vi "运维调试_总氮.vi"() -> ()   [LabVIEW 2016, in "总氮.lvlib"]
uses:
  <vilib>/Platform/TimedLoop/XDataNode/timing_clust.ctl
  <vilib>/Platform/TimedLoop/XDataNode/nitl_modes.ctl
  <vilib>/Platform/TimedLoop/XDataNode/wakeup.ctl
  <vilib>/Utility/miscctls.llb/LVPointTypeDef.ctl
  <vilib>/Platform/TimedLoop/XDataNode/XDataNode.xnode
  <vilib>/Platform/TimedLoop/XDataNode/XDNodeRunTimeDep.lvlib
  <vilib>/Utility/config.llb/NI_LVConfig.lvlib
panel:
  in  "总氮自动测试量程配置":T1
  out "温度2":sgl
  out "温度1":sgl
  out "ADC":sgl
  out "字符串":string
  out "固件版本号":string
  in  "数组":string[](array[string])
  in  "备用系数写入":bool
  in  "备用系数读取":bool
  in  "备用系数":T2
  in  "量程切换阈值写入":bool
  in  "量程切换阈值读取":bool
  in  "量程切换阈值":cluster{"阈值":dbl, "标液浓度":dbl}
  in  "参数下拉列表":enum16{"总磷", "总氮"}(ring)=enum."总氮"
  in  "量程下拉列表":enum16{"低量程", "高量程"}(ring)
  in  "测量模式下拉列表":enum16{"水样测量", "空白核查", "跨度核查", "标样核查", "加标回收"}(ring)
  in  "公式":cluster{"X^2":dbl, "X":dbl, "b":dbl}
  in  "写公式":bool
  in  "读公式":bool
  in  "精度":dbl=4.0
  in  "样品5 F0":dbl
  in  "样品5 F1":dbl
  in  "样品4 F1":dbl
  in  "样品4 F0":dbl
  in  "样品3 F0":dbl
  in  "样品3 F1":dbl
  in  "样品2 F0":dbl
  in  "样品2 F1":dbl
  in  "样品1 F1":dbl
  in  "样品1 F0":dbl
  in  "method":u16(ring) items=["最小二乘", "最小绝对残差", "Bisquare"]
  in  "模型":enum32{"线性", "多项式"}(ring)
  out "r^2":dbl format="%.7g"
  out "拟合公式":string
  in  "样品2启用":bool
  in  "样品5启用":bool
  in  "样品4启用":bool
  in  "样品3启用":bool
  in  "样品1启用":bool
  in  "标液浓度5":dbl
  out "测量吸光度5":dbl
  in  "标液浓度4":dbl
  out "测量吸光度4":dbl
  in  "标液浓度3":dbl
  out "测量吸光度3":dbl
  in  "标液浓度2":dbl
  out "测量吸光度2":dbl
  out "测量吸光度1":dbl
  in  "标液浓度1":dbl
  out "XY图":cluster{"X Values":dbl[], "Y Values":dbl[]}[](graph)
  in  "返回":bool
  in  "设置":bool
  out "序列号":string="序列号"
  out "总氮测量数据":T3(xcontrol)
  out "集成报警信息":string
  out "设置值":dbl
  out "定时启动":bool
  out "总磷总氮运行状态":T4(xcontrol)
  in  "停止":bool
  in  "手动启动":bool
  in  "单步测试":bool
  in  "总磷氨氮调试":u16[](xcontrol)
  out "F3":sgl format="%#.6f"
  out "F2":sgl format="%#.6f"
  out "F1":sgl format="%#.6f"
  out "F0":sgl format="%#.6f"
  out "多列列表框":i32(listbox)
  # "COM10"
  # "参数设置"
  # "标液浓度"
  # "F0"
  # "F1"
  # "吸光值显示"
  # "样品一"
  # "辅\n助\n计\n算\n区"
  # "样品二"
  # "样品三"
  # "样品四"
  # "样品五"
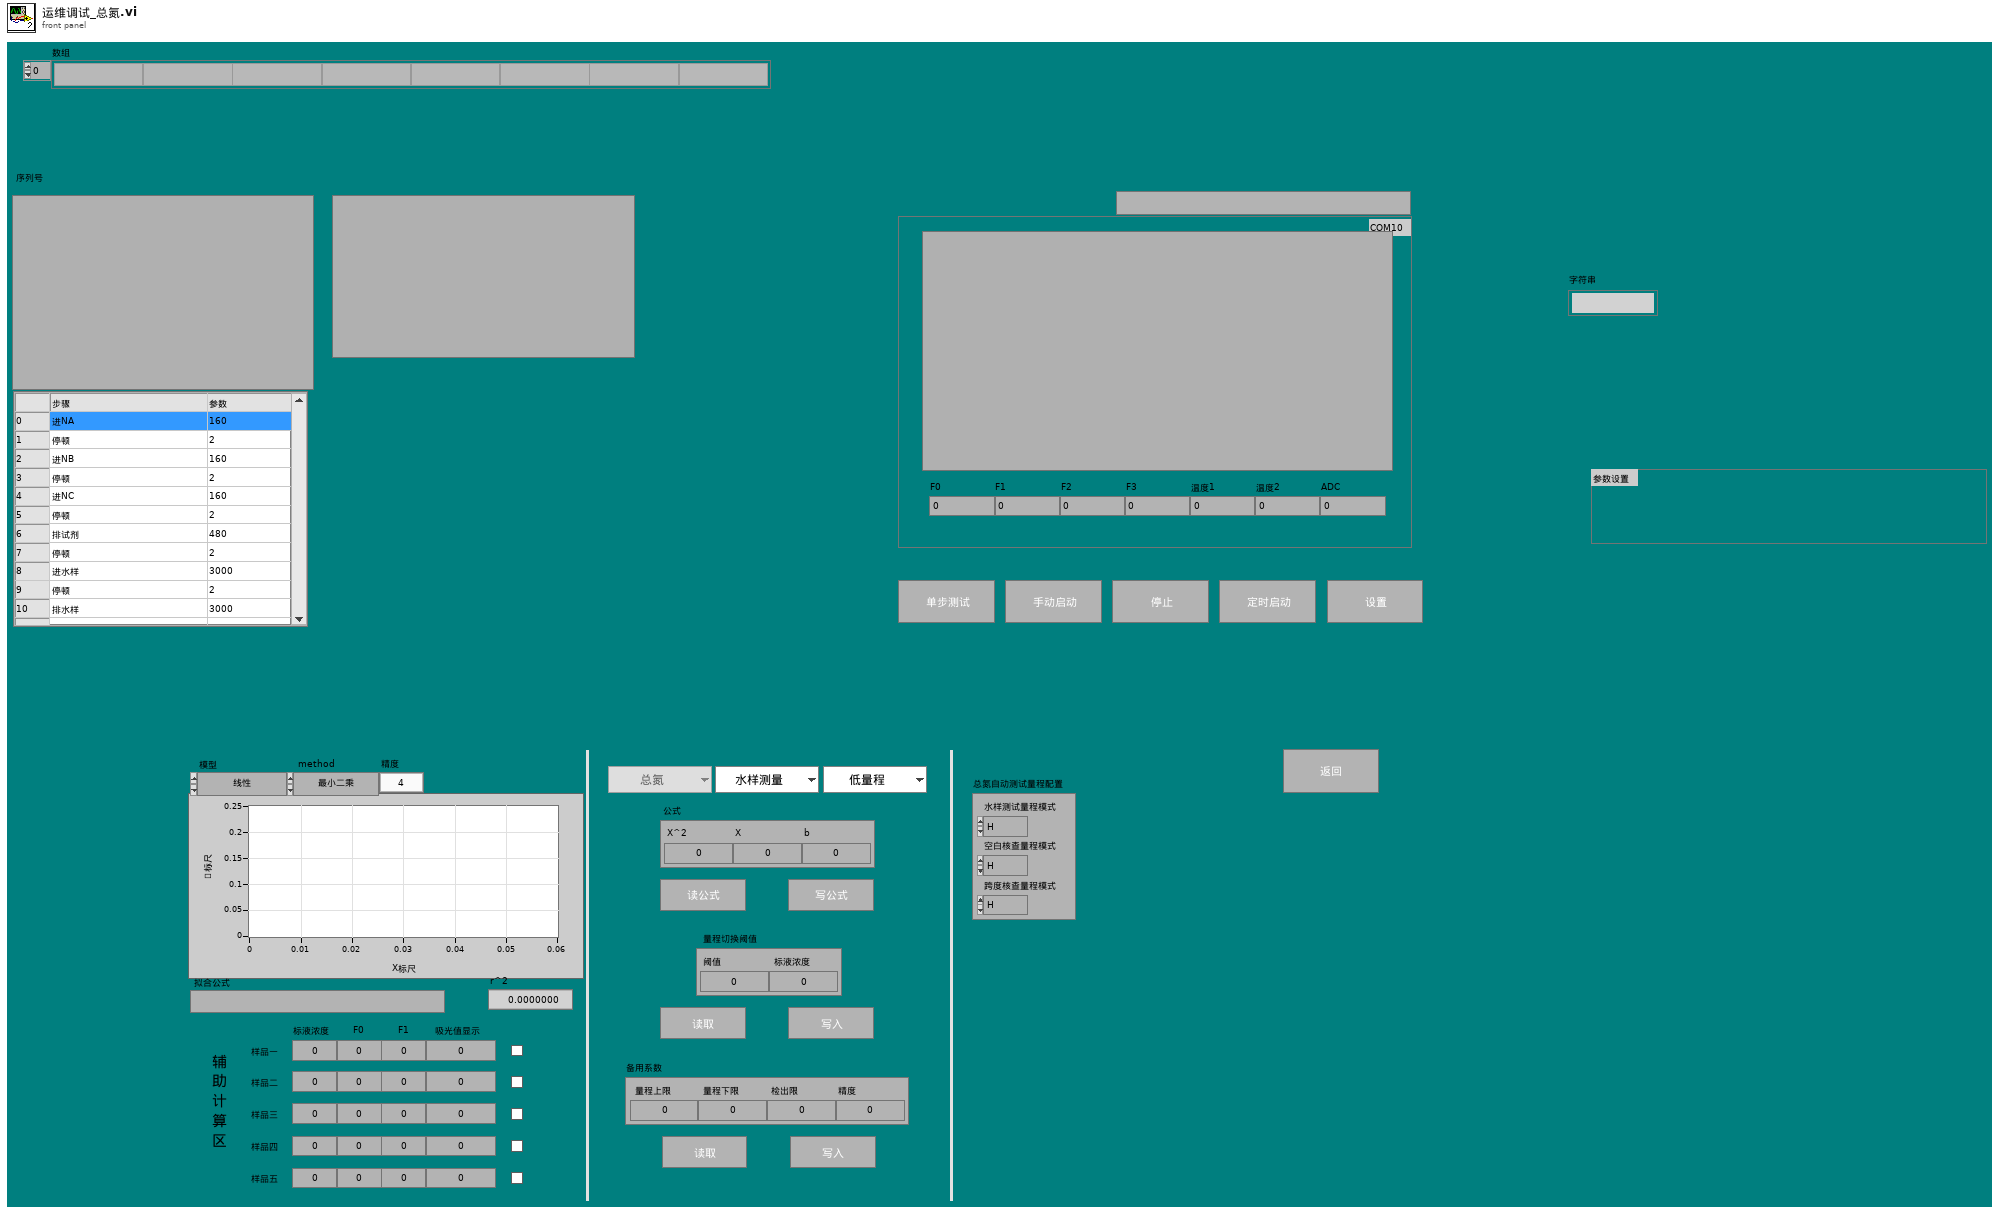
[diagram p1: front panel]
types:
  T1 = cluster{"水样测试量程模式":enum16{"H", "L", "AUTO"}, "空白核查量程模式":enum16{"H", "L", "AUTO"}, "跨度核查量程模式":enum16{"H", "L", "AUTO"}}
  T2 = cluster{"量程上限":dbl, "量程下限":dbl, "检出限":dbl, "精度":dbl}
  T3 = cluster{"flowid":u16, "测量精度":u16, "测量数据区":cluster{"因子编码":u32, "单位":u16, "标样参考值":sgl, "水样数据时间":timestamp, "水样实测值":sgl, "水样数据标识":string, "标样数据时间":timestamp, "标样实测值":sgl, "标样数据标识":string, "空白数据时间":timestamp, "空白实测值":sgl, "空白数据标识":string, "零点核查数据时间":timestamp, "零点核查实测值":sgl, "零点核查数据标识":string, "跨度核查数据时间":timestamp, "跨度核查实测值":sgl, "跨度核查数据标识":string, "加标回收数据时间":timestamp, "加标回收实测值":sgl, "加标回收数据标识":string, "平行样数据时间":timestamp, "平行样实测值":sgl, "平行样数据标识":string, "F0":sgl, "F1":sgl, "F2":sgl, "F3":sgl, "F4":sgl, "F5":sgl, "F6":sgl, "F7":sgl, "温度":sgl, "湿度":sgl, "X值":sgl}}
  T4 = cluster{"系统时间":timestamp, "工作状态":enum16{"空闲", "水样测试", "标样核查", "零点核查", "跨度核查", "空白测试", "平行样测试", "加标回收", "空白校准", "标样校准", "初始化（清洗）"}, "测量模式":enum16{"待机", "连续模式", "周期模式", "定点模式", "受控模式", "手动模式"}, "告警代码":enum16{"无告警", "缺试剂告警", "缺水样告警", "缺蒸馏水告警", "缺标液告警", "仪表漏液告警", "标定异常告警", "超量程告警", "加热异常", "低试剂预警", "超上限告警", "超下限告警", "仪表内部其他异常", "滴定异常告警", "电极异常告警", "量程切换告警", "参数设置告警", "PH电极电位异常", "电导率电极异常", "浊度光度异常", "溶解氧电极异常", "溶解氧光强异常", "温度异常告警", "PH异常告警", "溶解氧异常告警", "电导率异常告警", "浊度异常告警", "叶绿素异常告警", "藻密度异常告警", "蓝绿藻异常告警", "ORP异常告警", "氨氮异常告警", "清洁刷异常告警", "SD卡异常告警", "蓝牙异常告警", "Wifi异常告警", "流程异常告警"}, "故障代码":enum16{"无故障", "电机故障", "温度故障", "通讯故障", "滴定故障"}, "日志代码":u16, "软件版本":u16, "F0":sgl, "F1":sgl, "F2":sgl, "F3":sgl, "T":sgl, "H":sgl, "id":u16, "flowid":u16, "量程":u16, "总磷控温温度1":sgl, "营养盐控温温度2":sgl, "ADC":sgl}
  T5 = typedef "LVPointTypeDef.ctl" = cluster{"Horizontal":i16, "Vertical":i16}
  T6 = cluster{"因子编码":u32, "单位":u16, "标样参考值":sgl, "水样数据时间":timestamp, "水样实测值":sgl, "水样数据标识":string, "标样数据时间":timestamp, "标样实测值":sgl, "标样数据标识":string, "空白数据时间":timestamp, "空白实测值":sgl, "空白数据标识":string, "零点核查数据时间":timestamp, "零点核查实测值":sgl, "零点核查数据标识":string, "跨度核查数据时间":timestamp, "跨度核查实测值":sgl, "跨度核查数据标识":string, "加标回收数据时间":timestamp, "加标回收实测值":sgl, "加标回收数据标识":string, "平行样数据时间":timestamp, "平行样实测值":sgl, "平行样数据标识":string, "F0":sgl, "F1":sgl, "F2":sgl, "F3":sgl, "F4":sgl, "F5":sgl, "F6":sgl, "F7":sgl, "温度":sgl, "湿度":sgl, "X值":sgl}
  T7 = enum16{"空闲", "水样测试", "标样核查", "零点核查", "跨度核查", "空白测试", "平行样测试", "加标回收", "空白校准", "标样校准", "初始化（清洗）"}
  T8 = typedef "XDNodeRunTimeDep.lvlib/timing_clust.ctl" = cluster{"Expected End [f-1]":u64, "Actual End [f-1]":u64, "Finished Late? [f-1]":bool, "Expected End [i-1]":u64, "Actual End [i-1]":u64, "Finished Late? [i-1]":bool, "Expected Start [i]":u64, "Actual Start [i]":u64, "Expected Start [f]":u64, "Actual Start [f]":u64, "Source Name":string, "Structure Name":string, "Period":i64, "Deadline":i64, "Offset":i64, "Start":i64, "Priority":i32, "Timeout":i32, "Mode":T9, "Wakeup Reason":T10, "Error":errorcluster, "Source Type":string, "Secondary Source Type":string, "Global End Time":u64, "Global Start Time":u64, "Frame Duration":u64, "Iteration Duration":u64, "Assigned CPU":i32, "I/O Scan Engine Mode":u32}
  T9 = typedef "XDNodeRunTimeDep.lvlib/nitl_modes.ctl" = enum32{"No Change", "Process missed periods, maintain original phase", "Discard missed periods, maintain original phase", "Process missed periods, ignore original phase", "Discard missed periods, ignore original phase"}
  T10 = typedef "XDNodeRunTimeDep.lvlib/wakeup.ctl" = enum32{"Normal", "Aborted", "Asynchronous wakeup", "Timing source error", "Timed loop error", "Timeout"}
  T11 = cluster{"启动模式":enum16{"标液测量", "水样测量", "零液测量", "盲样测量", "加标回收"}, "启动参数":u16, "量程":enum16{"低量程", "高量程"}}
  T12 = cluster{"时间标识":timestamp, "设备":string, "日志信息":string, "流程参数":string}
  T13 = cluster{"时间标识":timestamp, "设备":string, "日志信息":string}
  T14 = enum16{"无告警", "缺试剂告警", "缺水样告警", "缺蒸馏水告警", "缺标液告警", "仪表漏液告警", "标定异常告警", "超量程告警", "加热异常", "低试剂预警", "超上限告警", "超下限告警", "仪表内部其他异常", "滴定异常告警", "电极异常告警", "量程切换告警", "参数设置告警", "PH电极电位异常", "电导率电极异常", "浊度光度异常", "溶解氧电极异常", "溶解氧光强异常", "温度异常告警", "PH异常告警", "溶解氧异常告警", "电导率异常告警", "浊度异常告警", "叶绿素异常告警", "藻密度异常告警", "蓝绿藻异常告警", "ORP异常告警", "氨氮异常告警", "清洁刷异常告警", "SD卡异常告警", "蓝牙异常告警", "Wifi异常告警", "流程异常告警"}
  T15 = typedef "LVRowAndColumnUnsignedTypeDef.ctl" = cluster{"Row":u32, "Column":u32}
  T16 = cluster{"站号":u16, "量程切换":enum32{"H", "L", "AUTO"}, "控制命令":enum16{"启动测量", "标样核查", "零点核查", "跨度核查", "空白测试", "平行样测试", "加标回收", "空白校准", "标样校准", "初始化（清洗）", "停止测试", "仪器重启", "校时", "模式设置", "测量间隔设置"}, "模式设置":enum16{"待机", "连续模式", "周期模式", "定点模式", "受控模式", "手动模式"}, "测量间隔":u16}
  T17 = typedef "NI_LVConfig.lvlib/Config Data RefNum.ctl" = refnum<k1>
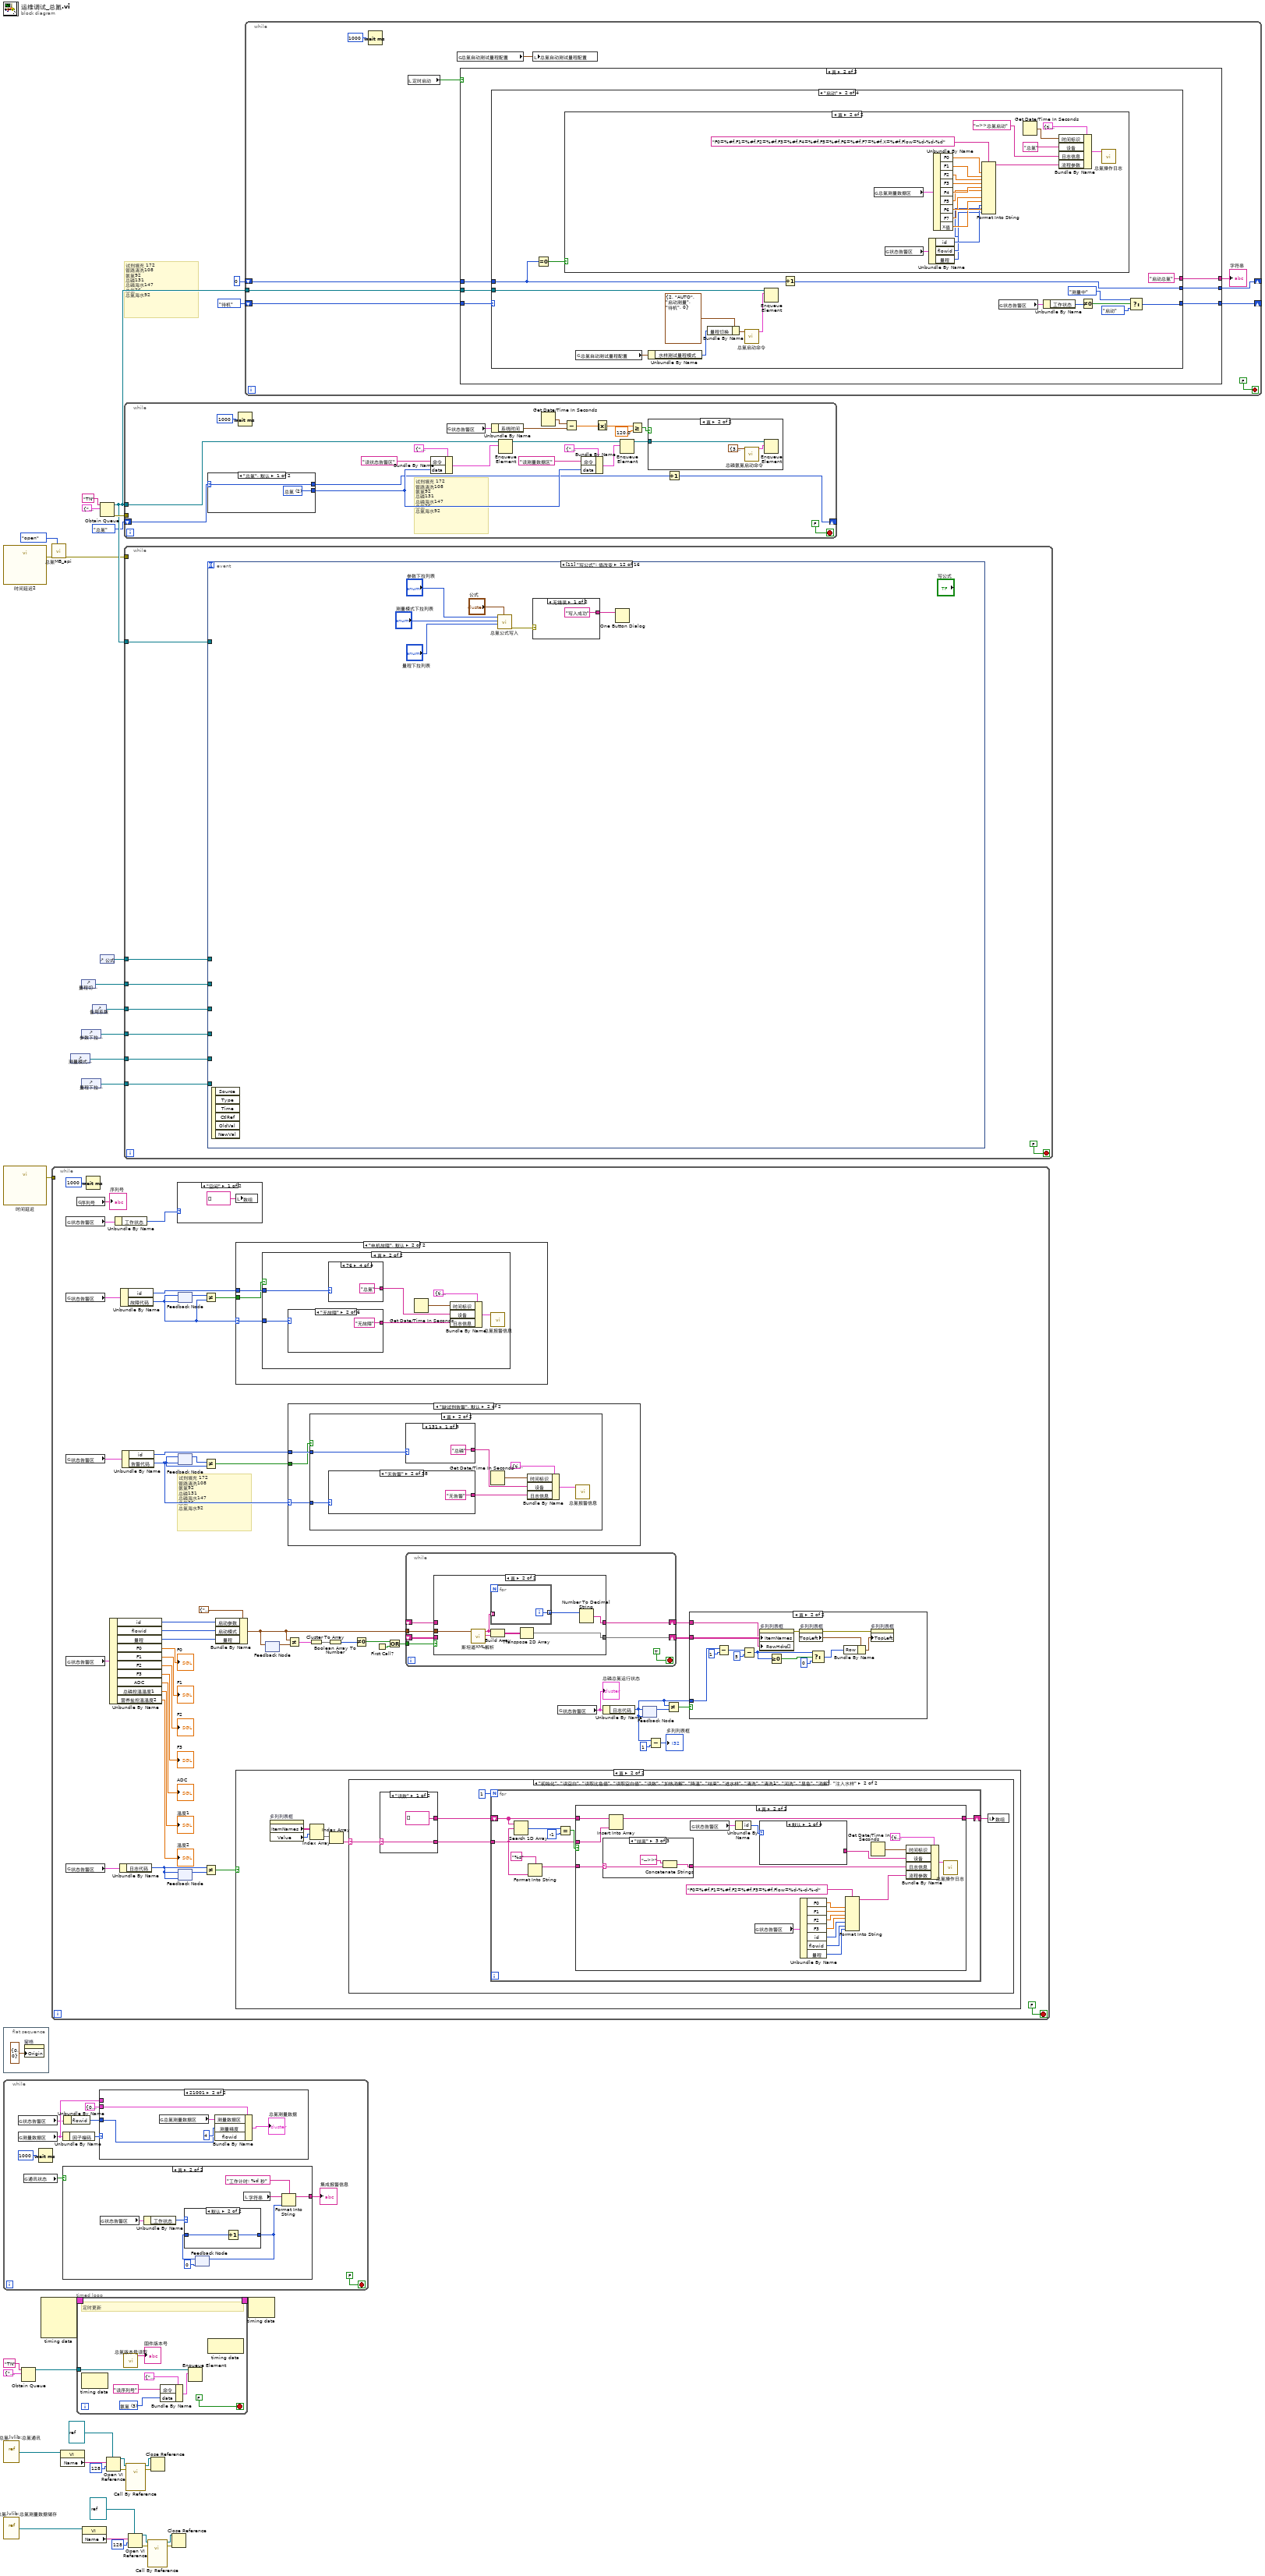
[diagram p0: block diagram]
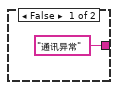
[diagram p2: hidden frame]
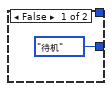
[diagram p5: hidden frame]
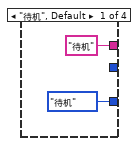
[diagram p6: hidden frame]
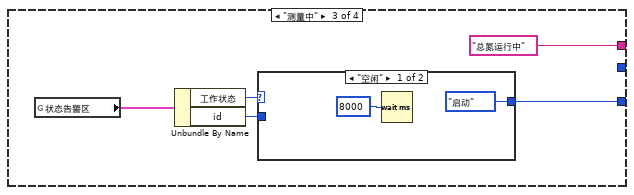
[diagram p8: hidden frame]
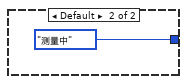
[diagram p9: hidden frame]
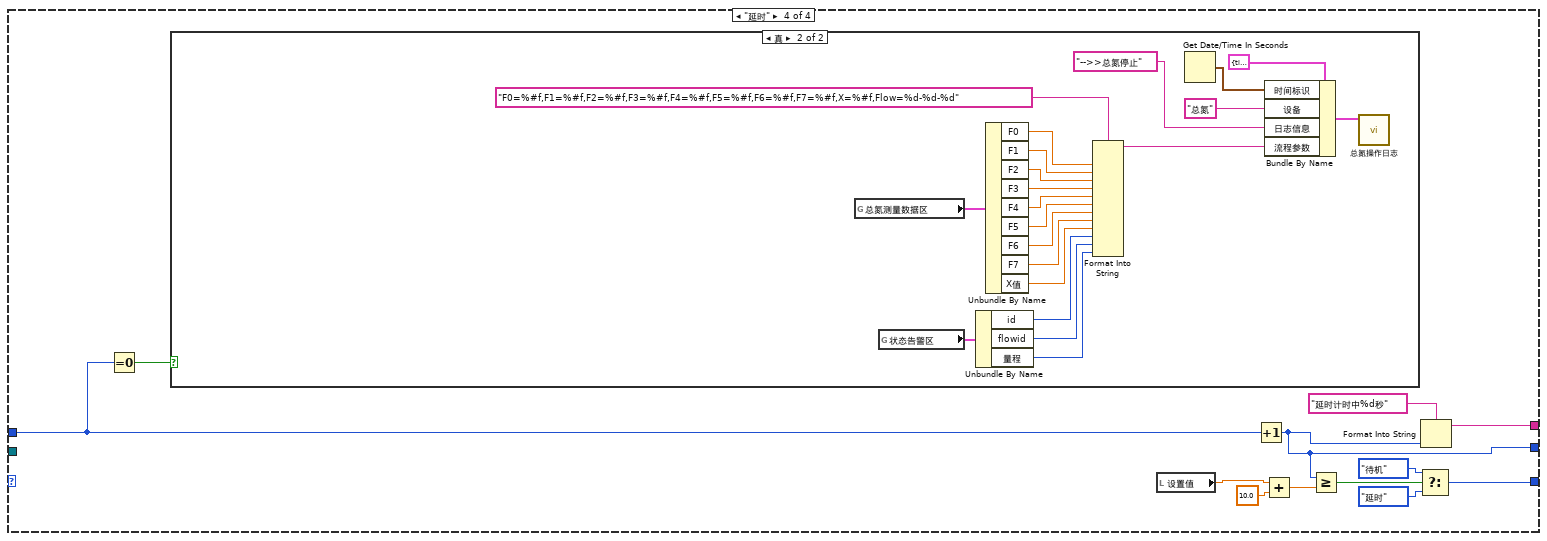
[diagram p10: hidden frame]
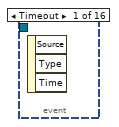
[diagram p12: hidden frame]
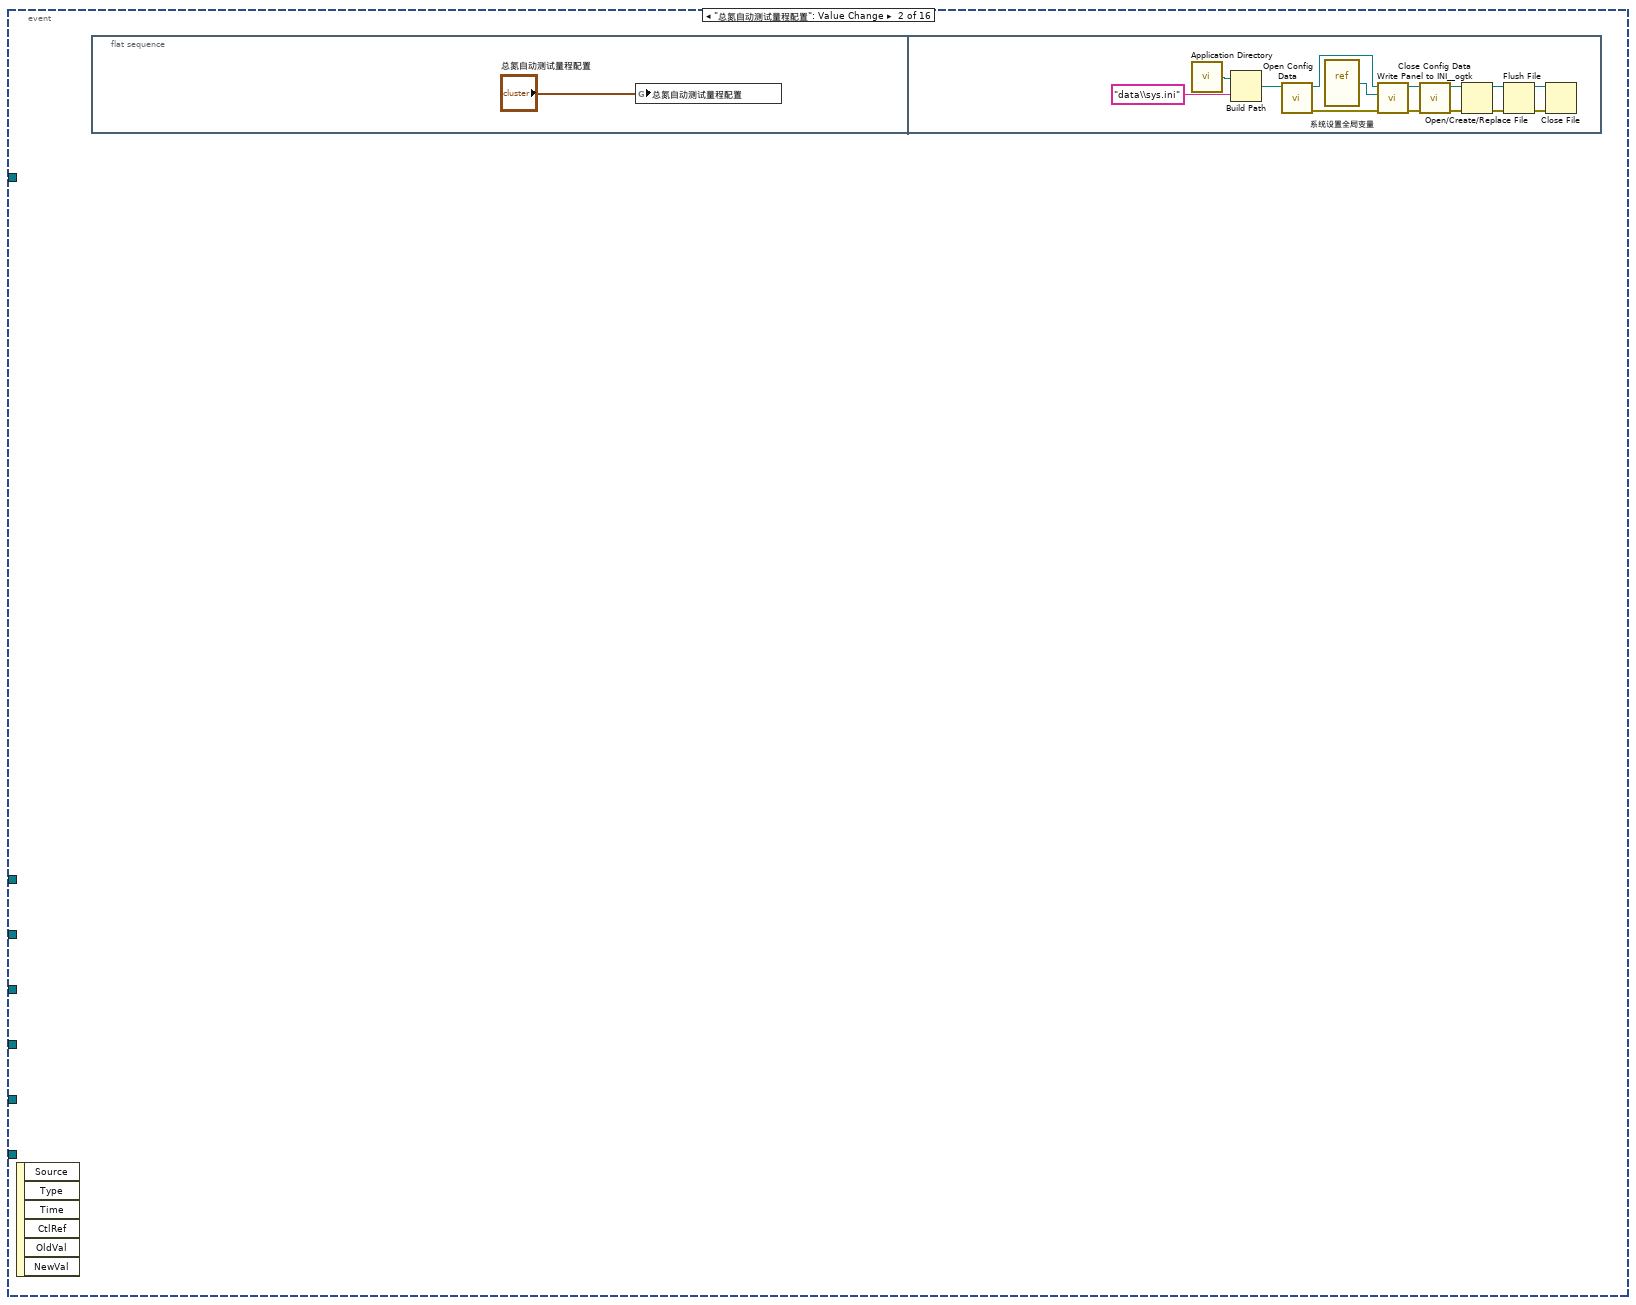
[diagram p13: hidden frame]
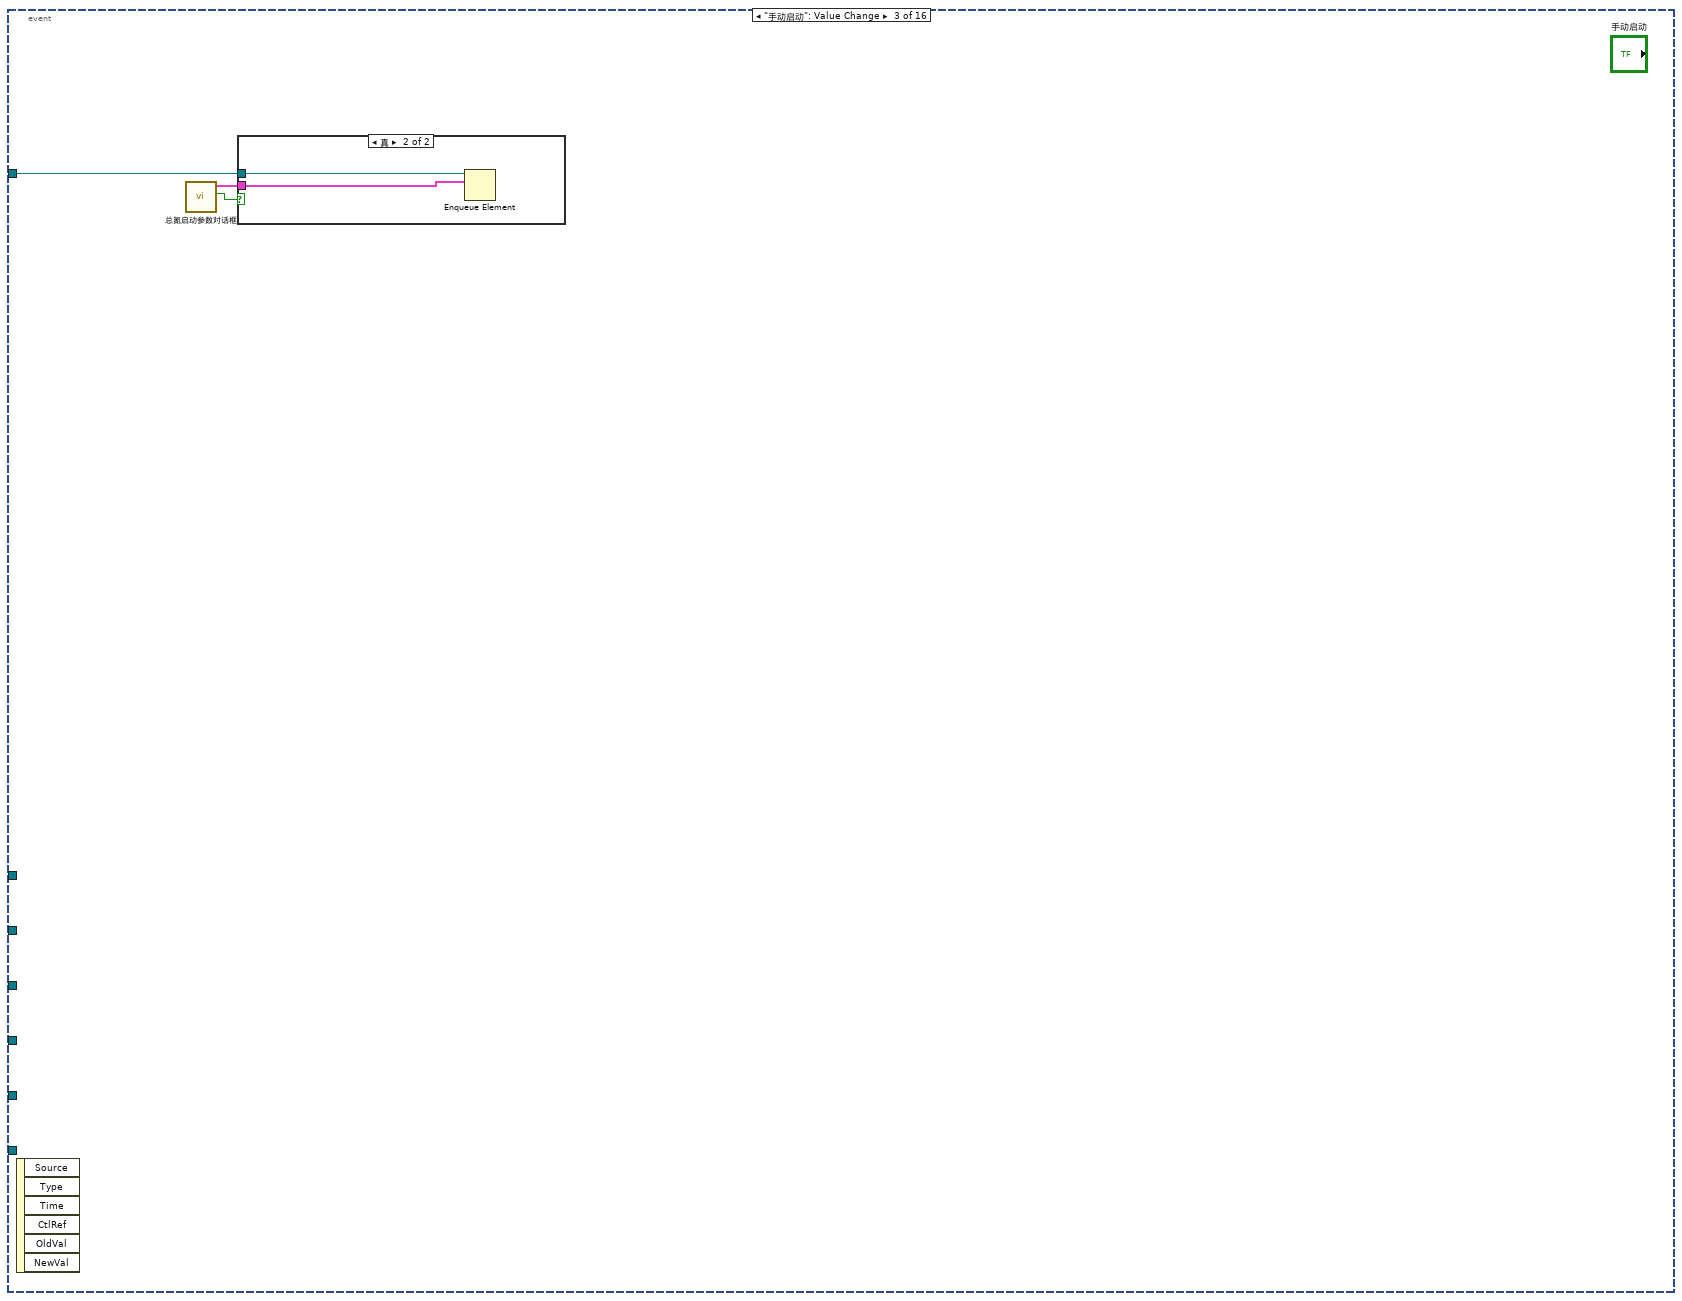
[diagram p14: hidden frame]
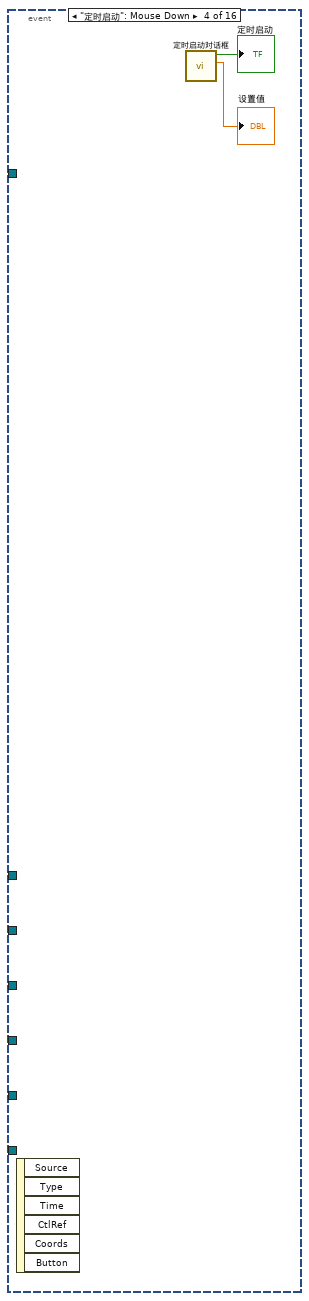
[diagram p16: hidden frame]
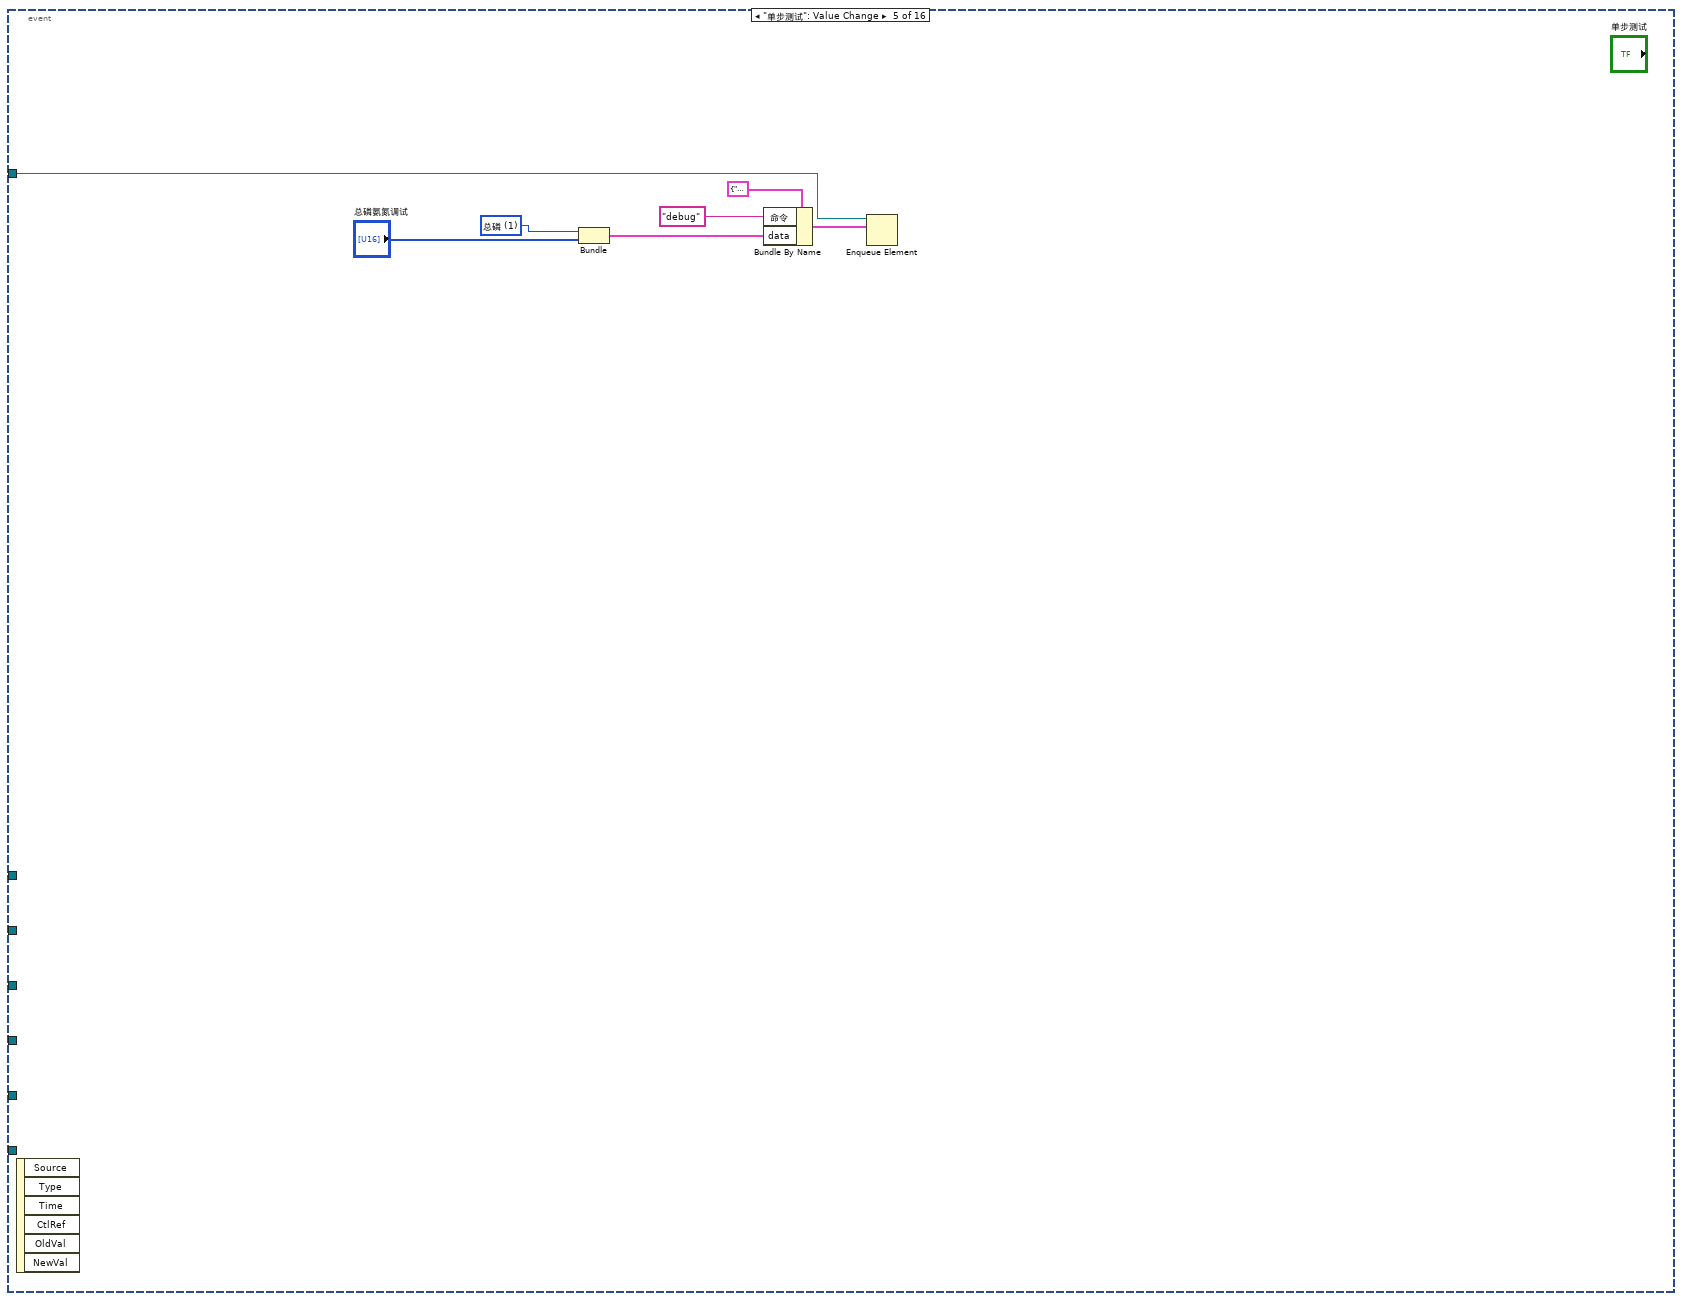
[diagram p17: hidden frame]
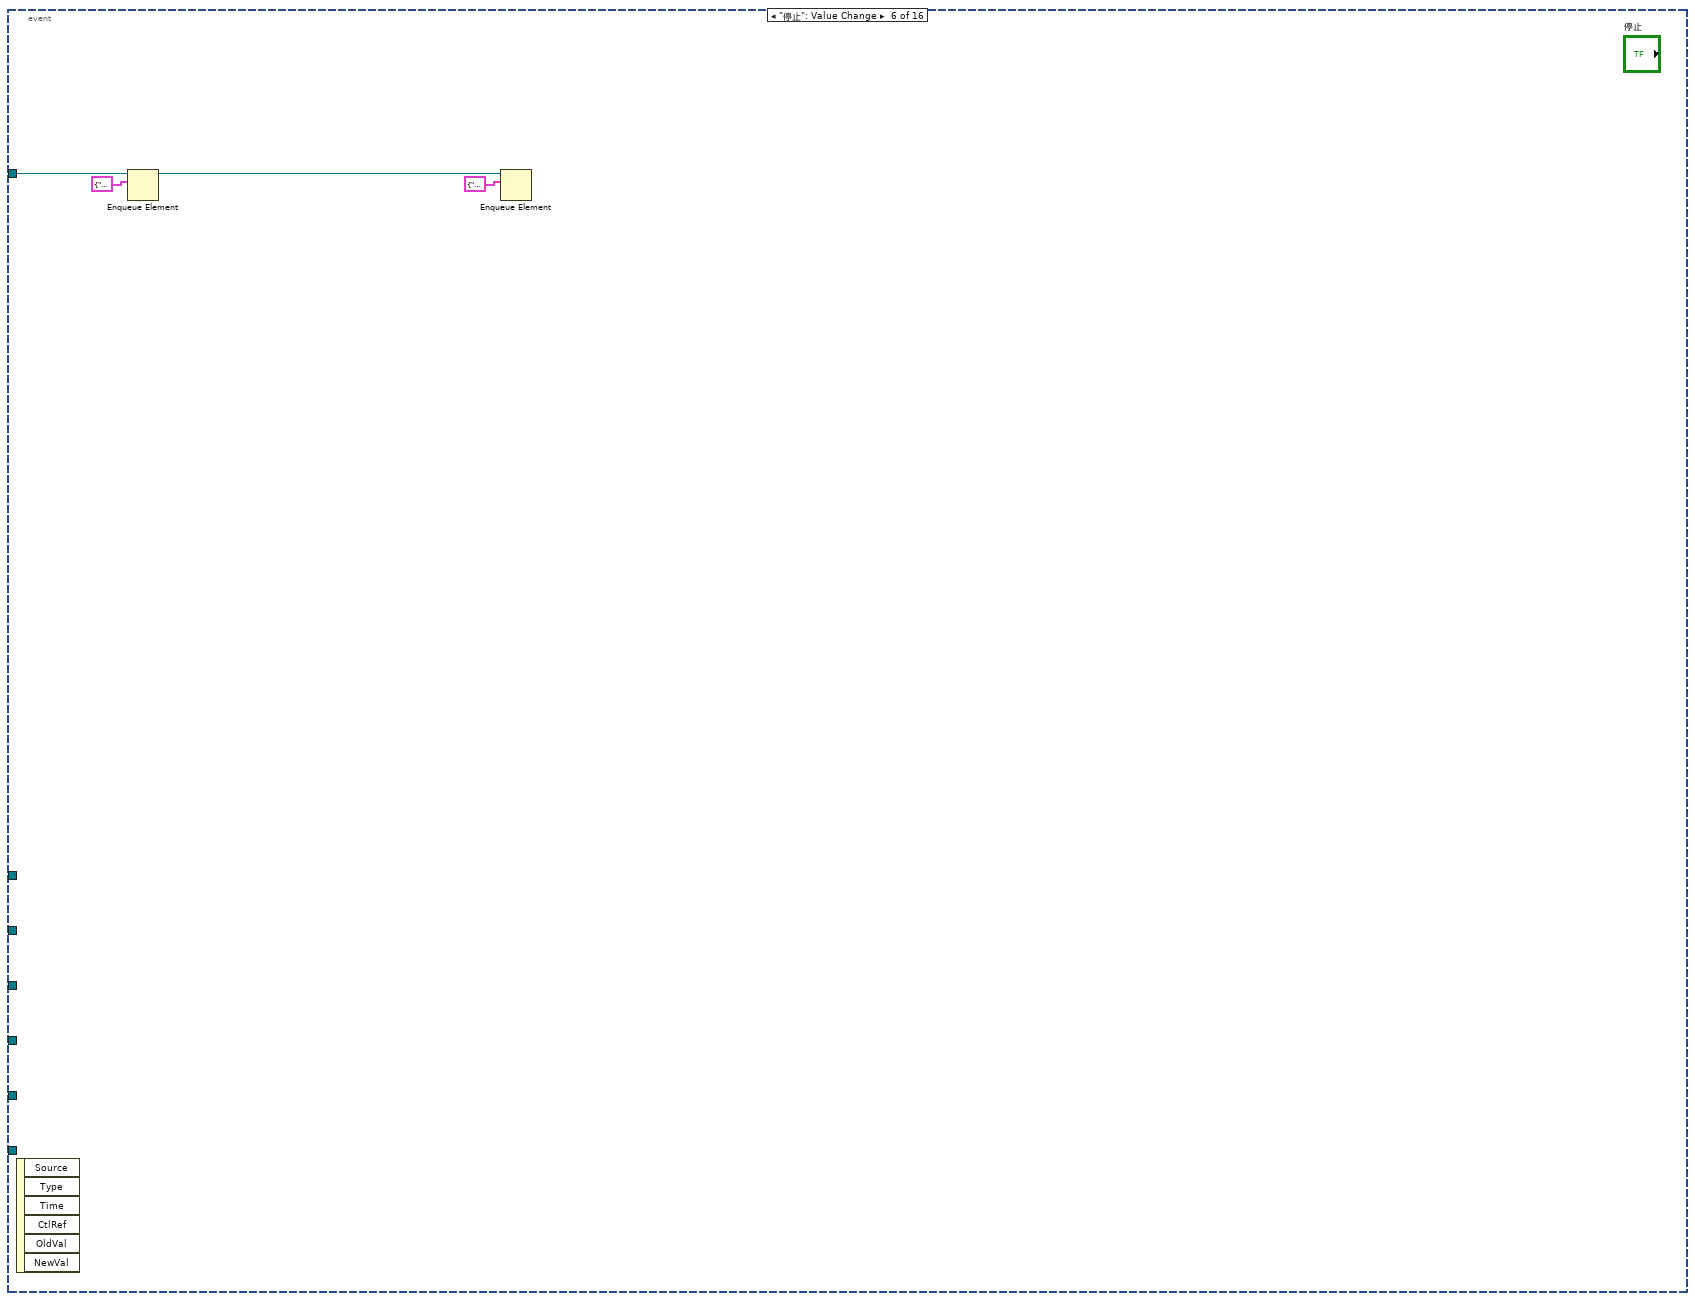
[diagram p18: hidden frame]
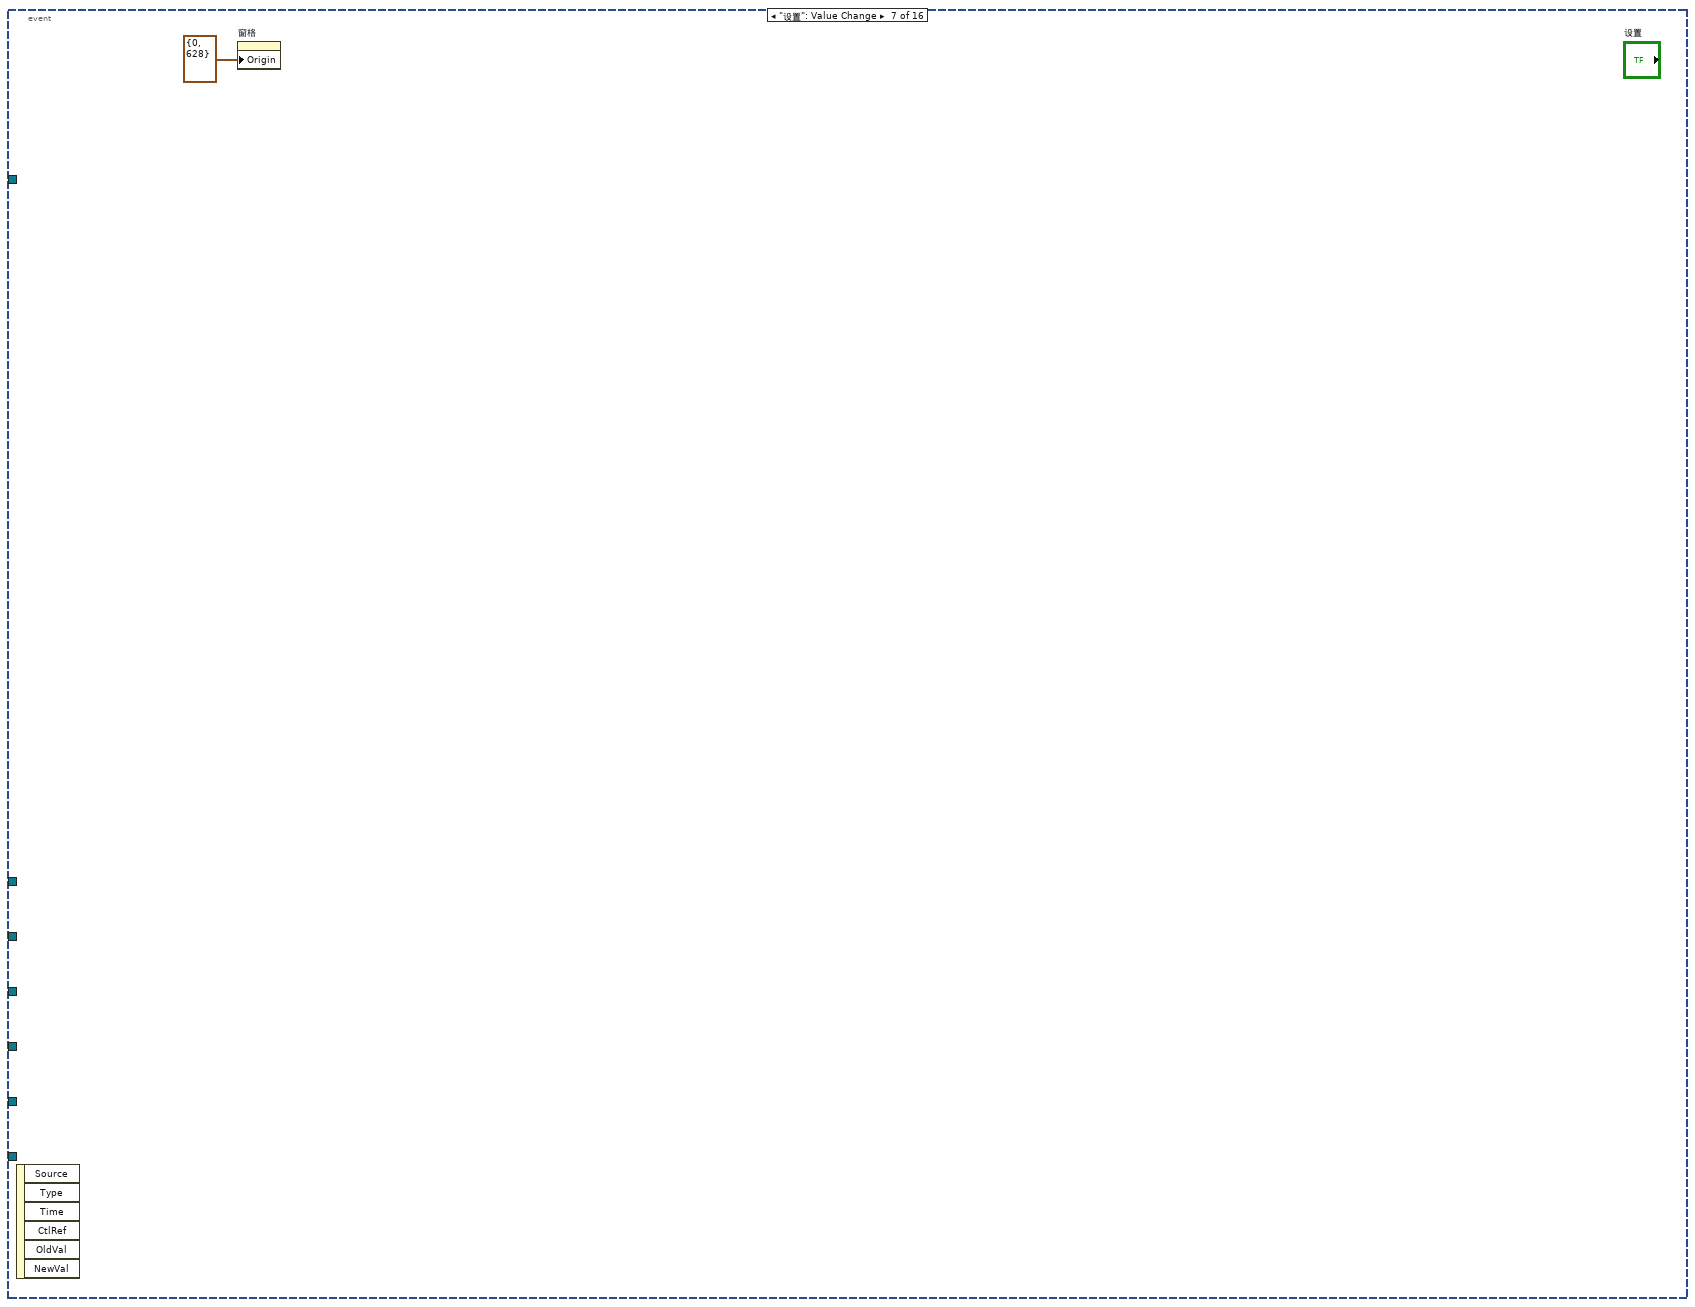
[diagram p19: hidden frame]
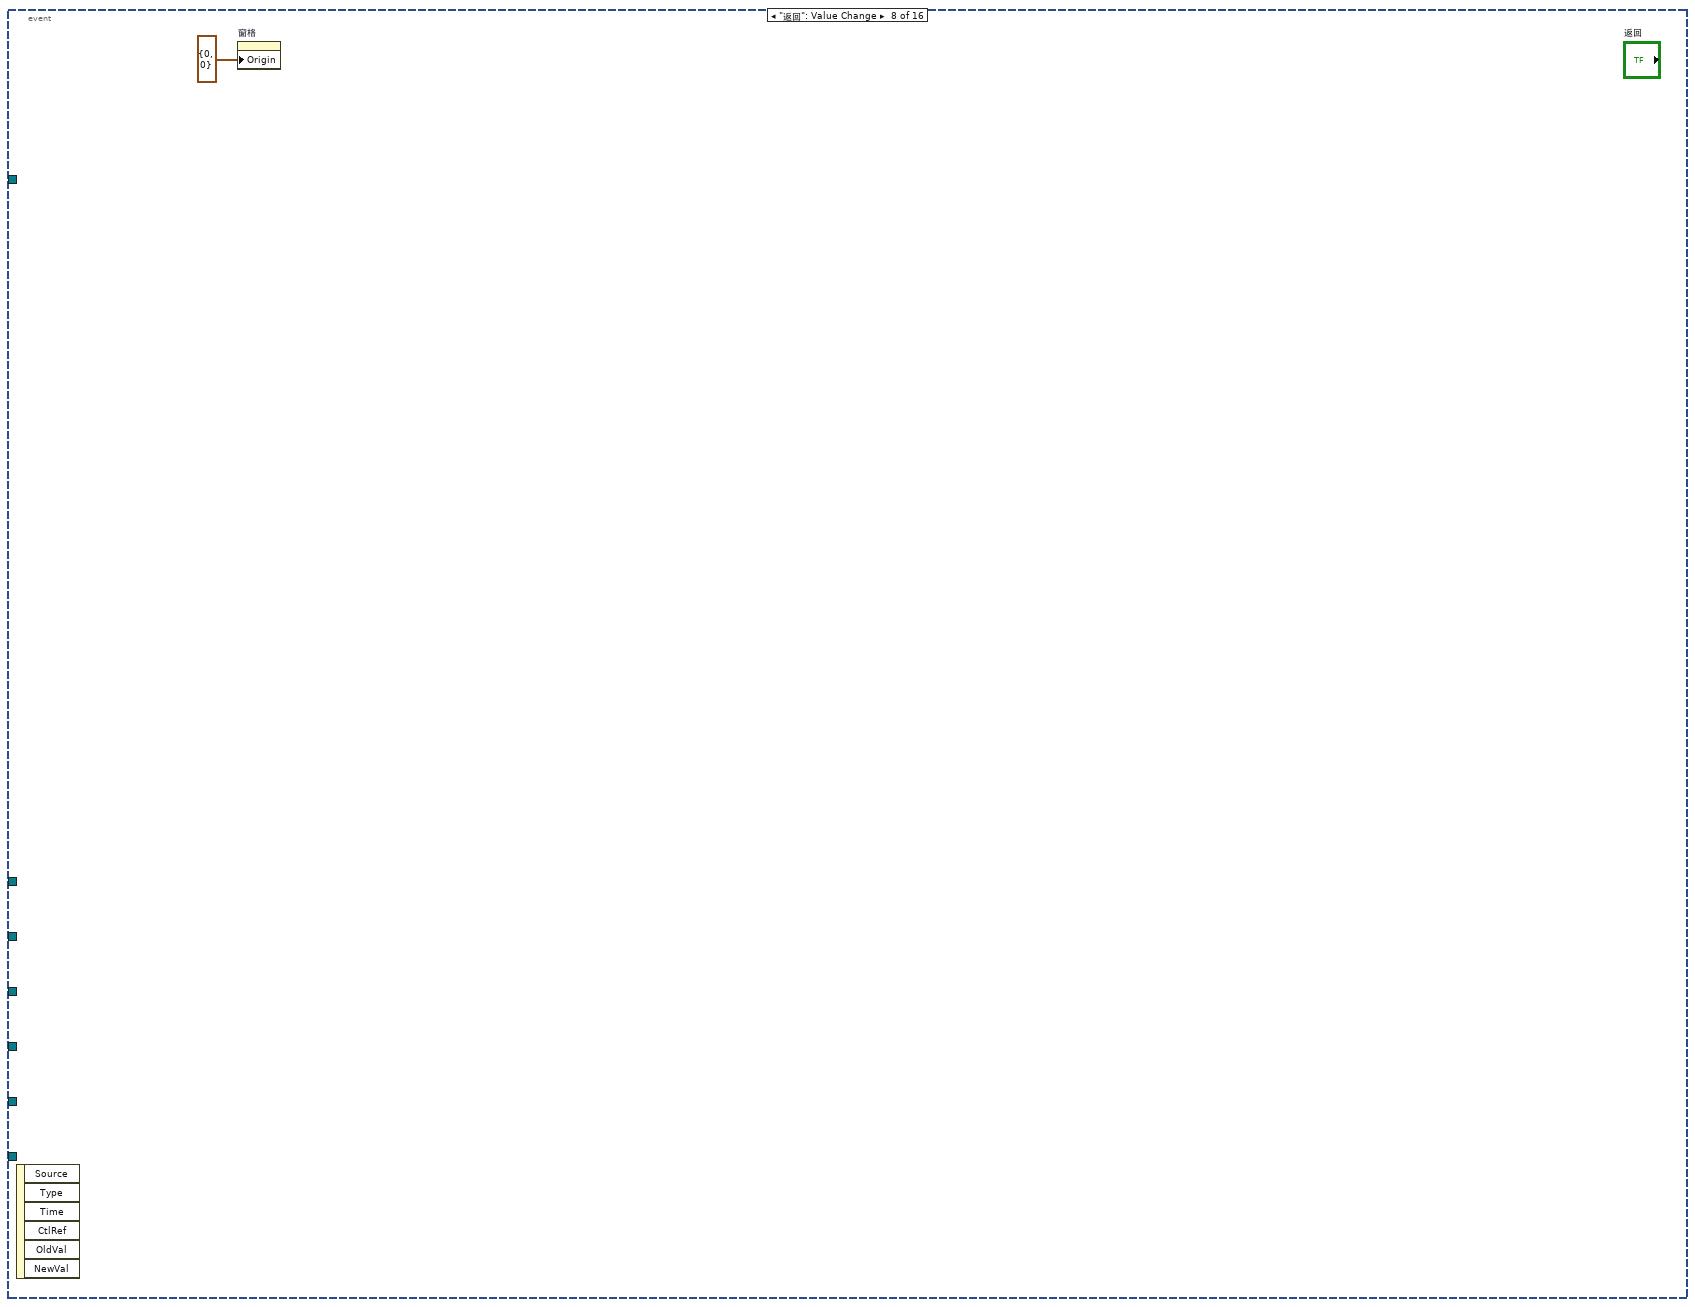
[diagram p20: hidden frame]
diagram:
  # "试剂填充 172 \n管路清洗108\n氨氮92\n总磷131\n总磷海水147\n总氮76\n总氮海水92"
  n1 = call "时间延迟2"() -> ("error out"=w1:errorcluster)  [unwired: 11 in]
  n2 = call "时间延迟"() -> ("error out"=w9:errorcluster)  [unwired: 11 in]
  n3 = flat-sequence {
    frame #0 {
      n4 = property on="窗格" class="Pane"("Origin"=T5 {"Horizontal"=0, "Vertical"=0} ("原点")) -> ()  [unwired: 2 in, 2 out]
    }
  }
  n5 = while {
    stop <- FALSE stop-if-true
    n6 = global read "VAR总氮全局变量.vi" "状态告警区"() -> (w42:T4)
    n7 = global read "VAR总氮全局变量.vi" "测量数据区"() -> (w46:T6)
    n8 = global read "VAR总氮全局变量.vi" "通讯状态"() -> (w44:bool)
    n9 = Wait (ms)(milliseconds to wait=u32 1000 ("等待时间（毫秒）")) -> ()  [unwired: 1 out]
    n10 = Unbundle By Name(w46) -> ("因子编码"=w45:u32)
    n11 = case shown="真" w44 {
      tunnel: ["通讯异常" ("集成报警信息") w51] -> w43
      frame False {
      }
      frame True {
        n12 = global read "VAR总氮全局变量.vi" "状态告警区"() -> (w57:T4)
        n13 = Unbundle By Name(w57) -> ("工作状态"=w56:T7)
        n14 = feedback #1(0) -> (w54:i32)
        n15 = case shown="默认" w56 {
          tunnel: w54 -> [_ w59]
          tunnel: [_ w58] -> w52
          frame "空闲" {
          }
          frame Default {
            n16 = Increment(x=w59) -> (x+1=w58:i32)
          }
        }
        n17 = feedback-in #1(w52) -> ()
        n18 = local read "字符串"() -> (w50:string)
        n19 = Format Into String(format string="工作计时: %d 秒" ("格式字符串"), initial string=w50, w52) -> (resulting string=w51:string)  [unwired: 1 in, 1 out]
      }
    }
    "集成报警信息" <- w43
    n20 = Unbundle By Name(w42) -> ("flowid"=w41:u16)
    n21 = case shown="21001" w45 {
      tunnel: w46 -> [_ _]
      tunnel: w41 -> [_ w63]
      tunnel: T3 {"flowid"=0, "测量精度"=0, "测量数据区"={"因子编码"=0, "单位"=0, "标样参考值"=0.0, "水样数据时间"=timestamp(0 s since 1904-01-01), "水样实测值"=0.0, "水样数据标识"="", "标样数据时间"=timestamp(0 s since 1904-01-01), "标样实测值"=0.0, "标样数据标识"="", "空白数据时间"=timestamp(0 s since 1904-01-01), "空白实测值"=0.0, "空白数据标识"="", "零点核查数据时间"=timestamp(0 s since 1904-01-01), "零点核查实测值"=0.0, "零点核查数据标识"="", "跨度核查数据时间"=timestamp(0 s since 1904-01-01), "跨度核查实测值"=0.0, "跨度核查数据标识"="", "加标回收数据时间"=timestamp(0 s since 1904-01-01), "加标回收实测值"=0.0, "加标回收数据标识"="", "平行样数据时间"=timestamp(0 s since 1904-01-01), "平行样实测值"=0.0, "平行样数据标识"="", "F0"=0.0, "F1"=0.0, "F2"=0.0, "F3"=0.0, "F4"=0.0, "F5"=0.0, "F6"=0.0, "F7"=0.0, "温度"=0.0, "湿度"=0.0, "X值"=0.0}} ("总氮测量数据") -> [_ w62]
      frame Default {
      }
      frame 21001 {
        n22 = global read "VAR总氮全局变量.vi" "总氮测量数据区"() -> (w61:T6)
        n23 = Bundle By Name(cluster=w62, "测量数据区"=w61, "测量精度"=u16 4, "flowid"=w63) -> (→"总氮测量数据":T3)
      }
    }
  }
  n24 = vi-ref "总氮.lvlib:总氮通讯.vi"() -> (w32:refnum<vi>)
  n25 = vi-ref "总氮.lvlib:总氮测量数据储存.vi"() -> (w24:refnum<vi>)
  n26 = Obtain Queue(name (unnamed)="TN" ("名称（未命名）"), element data type=cluster{"命令":string, "data":variant} {"命令"="", "data"=variant}) -> (queue out=w2:refnum<queue>)  [unwired: 3 in, 2 out]
  n27 = node-c288() -> (w6:T8)  [unwired: 4 in]
  n28 = call "总氮MB_api.vi"("STEP"=enum16{"open", "read", "write", "close"}."open", "Error in"=w1) -> ("error out"=w8:errorcluster)  [unwired: 7 in, 2 out]
  n29 = while {
    tunnel: w9 -> [_]
    stop <- FALSE stop-if-true
    # "试剂填充 172 \n管路清洗108\n氨氮92\n总磷131\n总磷海水147\n总氮76\n总氮海水92"
    n30 = global read "VAR总氮全局变量.vi" "状态告警区"() -> (w76:T4)
    n31 = global read "VAR总氮全局变量.vi" "状态告警区"() -> (w81:T4)
    n32 = global read "VAR总氮全局变量.vi" "状态告警区"() -> (w86:T4)
    n33 = global read "VAR总氮全局变量.vi" "状态告警区"() -> (w98:T4)
    n34 = global read "VAR总氮全局变量.vi" "状态告警区"() -> (w73:T4)
    n35 = global read "VAR总氮全局变量.vi" "序列号"() -> (→"序列号":string)
    n36 = Wait (ms)(milliseconds to wait=u32 1000 ("等待时间（毫秒）")) -> ()  [unwired: 1 out]
    n37 = Unbundle By Name(w98) -> ("id"=w95:u16, "flowid"=w97:u16, "量程"=w96:u16, "F0"=→"F0":sgl, "F1"=→"F1":sgl, "F2"=→"F2":sgl, "F3"=→"F3":sgl, "ADC"=→"ADC":sgl, "总磷控温温度1"=→"温度1":sgl, "营养盐控温温度2"=→"温度2":sgl)
    n38 = Unbundle By Name(w76) -> ("工作状态"=w75:T7)
    n39 = Unbundle By Name(w73) -> ("日志代码"=w72:u16)
    n40 = Unbundle By Name(w81) -> ("id"=w80:u16, "故障代码"=w77:enum16{"无故障", "电机故障", "温度故障", "通讯故障", "滴定故障"})
    n41 = Unbundle By Name(w86) -> ("id"=w85:u16, "告警代码"=w82:T14)
    n42 = case shown="\"空闲\"" w75 {
      frame "空闲" {
        n43 = local write "数组"(string[] [] ("数组")) -> ()
      }
      frame "水样测试", Default {
      }
    }
    n44 = feedback #2(w77) -> (w78:enum16{"无故障", "电机故障", "温度故障", "通讯故障", "滴定故障"})
    n45 = feedback-in #2(w77) -> ()
    n46 = feedback #3(w82) -> (w83:T14)
    n47 = feedback-in #3(w82) -> ()
    n48 = feedback #4(w72) -> (w74:u16)
    n49 = feedback-in #4(w72) -> ()
    n50 = Not Equal?(x=w78, y=w77) -> (x != y?=w79:bool)
    n51 = Not Equal?(x=w83, y=w82) -> (x != y?=w84:bool)
    n52 = Not Equal?(x=w72, y=w74) -> (x != y?=w71:bool)
    n53 = Bundle By Name(cluster=T11 {"启动模式"=enum."加标回收", "启动参数"=1, "量程"=enum."低量程"} ("参数簇"), "启动参数"=w95, "启动模式"=w97, "量程"=w96) -> (w88:T11)
    n54 = case shown="\"电机故障\", 默认" w77 {
      selector: w77 -> [_ w167]
      tunnel: w80 -> [_ w168]
      tunnel: w79 -> [_ w166]
      frame "无故障" {
      }
      frame "电机故障", Default {
        n55 = case shown="真" w166 {
          tunnel: w168 -> [_ w175]
          tunnel: w167 -> [_ w170]
          frame False {
          }
          frame True {
            n56 = case shown="\"无故障\"" w170 {
              selector: w170 -> [w177 _ _ _ _ _]
              tunnel: [w176 "无故障" "电机故障" "温度故障" "通讯故障" "滴定故障"] -> w169
              frame Default {
                n57 = Format Into String(format string="%d" ("格式字符串"), initial string="未知" ("工作状态"), w177) -> (resulting string=w176:string)  [unwired: 1 in, 1 out]
              }
              frame "无故障" {
              }
              frame "电机故障" {
              }
              frame "温度故障" {
              }
              frame "通讯故障" {
              }
              frame "滴定故障" {
              }
            }
            n58 = case shown="76" w175 {
              tunnel: [_ "总磷" ("table输入") "氨氮" ("table输入") "总氮" ("table输入")] -> w171
              frame Default {
              }
              frame 131 {
              }
              frame 92 {
              }
              frame 76 {
              }
            }
            n59 = Get Date/Time In Seconds() -> (seconds since 1Jan1904=w172:timestamp)
            n60 = Bundle By Name(cluster=T13 {"时间标识"=timestamp(0 s since 1904-01-01), "设备"="", "日志信息"=""} ("data in"), "时间标识"=w172, "设备"=w171, "日志信息"=w169) -> (w173:T13)
            n61 = call "总氮报警信息.vi"("data in"=w173) -> ()  [unwired: 11 in]
          }
        }
      }
    }
    n62 = case shown="真" w71 {
      frame False {
      }
      frame True {
        n63 = property on="多列列表框" class="MCListbox (严格)"() -> ("ItemNames"=w115:string[][], "Value"=w116:i32)  [unwired: 2 in, 2 out]
        n64 = Index Array(array=w115, index (row)=w116) -> (element=w114:string[])  [unwired: 1 in]
        n65 = Index Array(array=w114) -> (element=w113:string)  [unwired: 1 in]
        n66 = case shown="\"初始化\", \"读空白\", \"读取比色值\", \"读取空白值\", \"读数\", \"加热消解\", \"降温\", \"结束\", \"进水样\", \"清洗\", \"清洗1\", \"润洗\", \"显色\", \"消解\", \"注入水样\"" w113 {
          selector: w113 -> [_ w119]
          frame Default {
          }
          frame "初始化", "读空白", "读取比色值", "读取空白值", "读数", "加热消解", "降温", "结束", "进水样", "清洗", "清洗1", "润洗", "显色", "消解", "注入水样" {
            n67 = case shown="\"读数\"" w119 {
              selector: w119 -> [w123 w125]
              tunnel: [w123 w125] -> w118
              tunnel: [string[] [] ("数组") "数组"] -> w117
              frame "读数" {
              }
              frame Default {
              }
            }
            n68 = for {
              N: 1 -> [_]
              tunnel: w118 -> [w127]
              shift-right: [w126] -> w120
              shift-left: w117 -> [w128]
              n69 = Search 1D Array(1D array=w128, element=w127) -> (index of element=w131:i32)  [unwired: 1 in]
              n70 = Format Into String(format string="%s" ("格式字符串"), w127) -> (resulting string=w132:string)  [unwired: 2 in, 1 out]
              n71 = Equal?(x=w131, y=-1) -> (x = y?=w129:bool)
              n72 = case shown="真" w129 {
                tunnel: w132 -> [_ w136]
                tunnel: w128 -> [w134 w140]
                tunnel: w127 -> [_ w139]
                tunnel: [w134 w138] -> w126
                frame False {
                }
                frame True {
                  n73 = case shown="\"结束\"" w136 {
                    selector: w136 -> [w156 w159 w162]
                    tunnel: [w156 w158 w161] -> w135
                    frame Default {
                    }
                    frame "初始化" {
                      n74 = Concatenate Strings("-->>" ("字符串"), w159) -> (w158:string)
                    }
                    frame "结束" {
                      n75 = Concatenate Strings("-->>" ("字符串"), w162) -> (w161:string)
                    }
                  }
                  n76 = Insert Into Array(array=w140, new element=w139) -> (w138:string[])  [unwired: 1 in]
                  n77 = global read "VAR总氮全局变量.vi" "状态告警区"() -> (w155:T4)
                  n78 = Unbundle By Name(w155) -> ("id"=w154:u16)
                  n79 = global read "VAR总氮全局变量.vi" "状态告警区"() -> (w150:T4)
                  n80 = case shown="默认" w154 {
                    tunnel: [_ "总磷" ("table输入") "氨氮" ("table输入") "总氮" ("table输入")] -> w152
                    frame Default {
                    }
                    frame 131 {
                    }
                    frame 92 {
                    }
                    frame 76 {
                    }
                  }
                  n81 = Unbundle By Name(w150) -> ("F0"=w147:sgl, "F1"=w146:sgl, "F2"=w145:sgl, "F3"=w144:sgl, "id"=w143:u16, "flowid"=w142:u16, "量程"=w141:u16)
                  n82 = Format Into String(format string="F0=%#f,F1=%#f,F2=%#f,F3=%#f,Flow=%d-%-d-%-d" ("格式字符串"), w147, w146, w145, w144, w143, w142, w141) -> (resulting string=w148:string)  [unwired: 2 in, 1 out]
                  n83 = Get Date/Time In Seconds() -> (seconds since 1Jan1904=w151:timestamp)
                  n84 = Bundle By Name(cluster=T12 {"时间标识"=timestamp(0 s since 1904-01-01), "设备"="", "日志信息"="", "流程参数"=""} ("data in"), "时间标识"=w151, "设备"=w152, "日志信息"=w135, "流程参数"=w148) -> (w153:T12)
                  n85 = call "总氮操作日志.vi"("data in"=w153) -> ()  [unwired: 11 in]
                }
              }
            }
            n86 = local write "数组"(w120) -> ()
          }
        }
      }
    }
    n87 = feedback #5() -> (w104:T11)  [unwired: 1 in]
    n88 = feedback-in #5(w88) -> ()
    n89 = Not Equal?(x=w88, y=w104) -> (x != y?=w105:cluster{"启动模式":bool, "启动参数":bool, "量程":bool})
    n90 = case shown="\"缺试剂告警\", 默认" w82 {
      selector: w82 -> [_ w189]
      tunnel: w85 -> [_ w190]
      tunnel: w84 -> [_ w188]
      frame "无告警" {
      }
      frame "缺试剂告警", Default {
        n91 = case shown="真" w188 {
          tunnel: w190 -> [_ w197]
          tunnel: w189 -> [_ w191]
          frame False {
          }
          frame True {
            n92 = case shown="\"无告警\"" w191 {
              selector: w191 -> [w199 _ _ _ _ _ _ _ _ _ _ _ _ _ _ _ _ _ _ _ _ _ _ _ _ _ _ _ _ _ _ _ _ _ _ _ _ _]
              tunnel: [w198 "无告警" "缺试剂告警" "缺水样告警" "缺蒸馏水告警" "缺标液告警" "仪表漏液告警" "标定异常告警" "超量程告警" "加热异常" "低试剂预警" "超上限告警" "超下限告警" "仪表内部其他异常" "滴定异常告警" "电极异常告警" "量程切换告警" "参数设置告警" "PH电极电位异常" "电导率电极异常" "浊度光度异常" "溶解氧电极异常" "溶解氧光强异常" "温度异常告警" "PH异常告警" "溶解氧异常告警" "电导率异常告警" "浊度异常告警" "叶绿素异常告警" "藻密度异常告警" "蓝绿藻异常告警" "ORP异常告警" "氨氮异常告警" "清洁刷异常告警" "SD卡异常告警" "蓝牙异常告警" "WiFi异常告警" "流程异常告警"] -> w192
              frame Default {
                n93 = Format Into String(format string="%d" ("格式字符串"), initial string="未知" ("工作状态"), w199) -> (resulting string=w198:string)  [unwired: 1 in, 1 out]
              }
              frame "无告警" {
              }
              frame "缺试剂告警" {
              }
              frame "缺水样告警" {
              }
              frame "缺蒸馏水告警" {
              }
              frame "缺标液告警" {
              }
              frame "仪表漏液告警" {
              }
              frame "标定异常告警" {
              }
              frame "超量程告警" {
              }
              frame "加热异常" {
              }
              frame "低试剂预警" {
              }
              frame "超上限告警" {
              }
              frame "超下限告警" {
              }
              frame "仪表内部其他异常" {
              }
              frame "滴定异常告警" {
              }
              frame "电极异常告警" {
              }
              frame "量程切换告警" {
              }
              frame "参数设置告警" {
              }
              frame "PH电极电位异常" {
              }
              frame "电导率电极异常" {
              }
              frame "浊度光度异常" {
              }
              frame "溶解氧电极异常" {
              }
              frame "溶解氧光强异常" {
              }
              frame "温度异常告警" {
              }
              frame "PH异常告警" {
              }
              frame "溶解氧异常告警" {
              }
              frame "电导率异常告警" {
              }
              frame "浊度异常告警" {
              }
              frame "叶绿素异常告警" {
              }
              frame "藻密度异常告警" {
              }
              frame "蓝绿藻异常告警" {
              }
              frame "ORP异常告警" {
              }
              frame "氨氮异常告警" {
              }
              frame "清洁刷异常告警" {
              }
              frame "SD卡异常告警" {
              }
              frame "蓝牙异常告警" {
              }
              frame "Wifi异常告警" {
              }
              frame "流程异常告警" {
              }
            }
            n94 = case shown="131" w197 {
              tunnel: ["总磷" ("table输入") "氨氮" ("table输入") "总氮" ("table输入")] -> w193
              frame 131 {
              }
              frame 92 {
              }
              frame 76, Default {
              }
            }
            n95 = Get Date/Time In Seconds() -> (seconds since 1Jan1904=w194:timestamp)
            n96 = Bundle By Name(cluster=T13 {"时间标识"=timestamp(0 s since 1904-01-01), "设备"="", "日志信息"=""} ("data in"), "时间标识"=w194, "设备"=w193, "日志信息"=w192) -> (w195:T13)
            n97 = call "总氮报警信息.vi"("data in"=w195) -> ()  [unwired: 11 in]
          }
        }
      }
    }
    n98 = Cluster To Array(cluster=w105) -> (array=w106:bool[])
    n99 = Boolean Array To Number(Boolean array=w106) -> (number=w107:u32)
    n100 = Not Equal To 0?(x=w107) -> (x != 0?=w100:bool)
    n101 = First Call?() -> (First Call?: T/F=w101:bool)
    n102 = Or(x=w100, y=w101) -> (x .or. y?=w99:bool)
    n103 = while {
      tunnel: w99 -> [w248]
      tunnel: w88 -> [w247]
      shift-right: [w246] -> w103
      shift-left: _ -> [w242]
      shift-right: [w245] -> w102
      shift-left: _ -> [w243]
      stop <- TRUE stop-if-true
      n104 = case shown="真" w248 {
        tunnel: [w250 w257] -> w245
        tunnel: [w249 w256] -> w246
        tunnel: w247 -> [_ w251]
        tunnel: w243 -> [w250 _]
        tunnel: w242 -> [w249 _]
        frame False {
        }
        frame True {
          n105 = call "斯坦道XML解析.vi"("参数簇"=w251) -> ("步骤时间"=w252:string[], "步骤名"=w254:string[])  [unwired: 9 in]
          n106 = for {
            tunnel: w254 -> [_] mode=indexing
            tunnel: [w258] -> w255 mode=indexing
            i -> [w258]
          }
          n107 = Build Array(w254, w252) -> (w253:string[][])
          n108 = Transpose 2D Array(2D array=w253) -> (transposed array=w256:string[][])
          n109 = Number To Decimal String(number=w255) -> (decimal integer string=w257:string[])  [unwired: 1 in]
        }
      }
    }
    n110 = global read "VAR总氮全局变量.vi" "状态告警区"() -> (w89:T4)
    "总磷总氮运行状态" <- w89
    n111 = Unbundle By Name(w89) -> ("日志代码"=w69:u16)
    n112 = feedback-in #6(w69) -> ()
    n113 = feedback #6(w69) -> (w109:u16)
    n114 = Subtract(x=w69, y=1) -> (x-y=→"多列列表框":i32)
    n115 = Not Equal?(x=w69, y=w109) -> (x != y?=w108:bool)
    n116 = case shown="真" w108 {
      tunnel: w69 -> [_ w261]
      tunnel: w103 -> [_ w268]
      tunnel: w102 -> [_ w267]
      frame False {
      }
      frame True {
        n117 = Subtract(x=w261, y=1) -> (x-y=w259:i32)
        n118 = Subtract(x=w259, y=5) -> (x-y=w263:i32)
        n119 = property on="多列列表框" class="MCListbox (严格)"("ItemNames"=w268, "RowHdrs[]"=w267) -> (error out=w269:errorcluster)  [unwired: 2 in, 1 out]
        n120 = Greater Or Equal To 0?(x=w263) -> (x >= 0?=w262:bool)
        n121 = property on="多列列表框" class="MCListbox (严格)"(error in=w269) -> (error out=w270:errorcluster, "TopLeft"=w271:T15)  [unwired: 1 in, 1 out]
        n122 = Select(t=w263, s=w262, f=0) -> (s? t:f=w264:i32)
        n123 = Bundle By Name(cluster=w271, "Row"=w264) -> (w272:T15)
        n124 = property on="多列列表框" class="MCListbox (严格)"(error in=w270, "TopLeft"=w272) -> ()  [unwired: 1 in, 2 out]
      }
    }
  }
  n125 = property class="VI"(reference=w32) -> ("Name"=w31:string)  [unwired: 1 in, 2 out]
  n126 = control-ref of="测量模式下拉列表"() -> (w13:refnum<vi>)
  n127 = timed-loop {
    timing: w6 -> [_]
    timing-out: [_] -> w5
    tunnel: w2 -> [w275]
    stop <- FALSE stop-if-true
    w276 = u16 3 items=["总磷"=1, "氨氮"=3] ("站号")
    # "定时更新"
    n128 = node-c288() -> ()  [unwired: 1 in, 1 out]
    n129 = call "总氮版本号读取.vi"() -> ("固件版本号"=→"固件版本号":string)  [unwired: 11 in]
    n130 = Bundle By Name(cluster=cluster{"命令":string, "data":variant} {"命令"="", "data"=variant} ("元素"), "命令"="读序列号", "data"=w276) -> (w274:cluster{"命令":string, "data":variant})
    n131 = Enqueue Element(queue=w275, element=w274) -> ()  [unwired: 2 in, 3 out]
    n132 = node-c288() -> ()  [unwired: 1 in, 1 out]
  }
  n133 = control-ref of="量程切换阈值"() -> (w11:refnum<vi>)
  n134 = control-ref of="参数下拉列表"() -> (w14:refnum<vi>)
  n135 = control-ref of="量程下拉列表"() -> (w15:refnum<vi>)
  n136 = property class="VI"(reference=w24) -> ("Name"=w17:string)  [unwired: 1 in, 2 out]
  n137 = control-ref of="备用系数"() -> (w10:refnum<vi>)
  n138 = Obtain Queue(name (unnamed)="TN" ("名称（未命名）"), element data type=cluster{"命令":string, "data":variant} {"命令"="", "data"=variant}) -> (queue out=w35:refnum<queue>, error out=w36:errorcluster)  [unwired: 3 in, 1 out]
  n139 = control-ref of="公式"() -> (w12:refnum<vi>)
  n140 = Open VI Reference(type specifier VI Refnum (for type only)=refnum<vi> refnum, vi path=w31, options=128 ("选项")) -> (vi reference=w29:refnum<vi>, error out=w27:errorcluster)  [unwired: 3 in]
  n141 = while {
    tunnel: w35 -> [w298]
    tunnel: w36 -> [_]
    shift-right: [w290] -> _
    shift-left: enum16{"总磷", "总氮"}."总氮" ("枚举") -> [w292]
    stop <- FALSE stop-if-true
    # "试剂填充 172 \n管路清洗108\n氨氮92\n总磷131\n总磷海水147\n总氮76\n总氮海水92"
    n142 = case shown="\"总氮\", 默认" w292 {
      selector: w292 -> [w307 w309]
      tunnel: [w308 w310] -> w293
      tunnel: [w307 w309] -> w291
      frame "总氮", Default {
        w308 = u16 2 items=["总磷"=1, "总氮"=2] ("站号")
      }
      frame "总磷" {
        w310 = u16 1 items=["总磷"=1, "氨氮"=3] ("站号")
      }
    }
    n143 = Wait (ms)(milliseconds to wait=u32 1000 ("等待时间（毫秒）")) -> ()  [unwired: 1 out]
    n144 = Bundle By Name(cluster=cluster{"命令":string, "data":variant} {"命令"="", "data"=variant} ("元素"), "命令"="读状态告警区", "data"=w293) -> (w300:cluster{"命令":string, "data":variant})
    n145 = global read "VAR总氮全局变量.vi" "状态告警区"() -> (w282:T4)
    n146 = Unbundle By Name(w282) -> ("系统时间"=w289:timestamp)
    n147 = Enqueue Element(queue=w298, element=w300) -> (queue out=w294:refnum<queue>)  [unwired: 2 in, 2 out]
    n148 = Get Date/Time In Seconds() -> (seconds since 1Jan1904=w288:timestamp)
    n149 = Subtract(x=w288, y=w289) -> (x-y=w287:dbl)
    n150 = Bundle By Name(cluster=cluster{"命令":string, "data":variant} {"命令"="", "data"=variant} ("元素"), "命令"="读测量数据区", "data"=w293) -> (w296:cluster{"命令":string, "data":variant})
    n151 = Absolute Value(x=w287) -> (abs(x)=w286:dbl)
    n152 = Enqueue Element(queue=w294, element=w296) -> (queue out=w283:refnum<queue>)  [unwired: 2 in, 2 out]
    n153 = Greater Or Equal?(x=w286, y=120.0) -> (x >= y?=w284:bool)
    n154 = case shown="真" w284 {
      tunnel: w283 -> [_ w305]
      frame False {
      }
      frame True {
        n155 = call "总磷氨氮启动命令.vi"("参数"=T16 {"站号"=3, "量程切换"=enum."AUTO", "控制命令"=enum."校时", "模式设置"=enum."待机", "测量间隔"=0}) -> ("启动命令"=w304:cluster{"命令":string, "data":variant})  [unwired: 10 in]
        n156 = Enqueue Element(queue=w305, element=w304) -> ()  [unwired: 2 in, 3 out]
      }
    }
    n157 = Increment(x=w291) -> (x+1=w290:enum16{"总磷", "总氮"})
  }
  n158 = while {
    tunnel: w35 -> [w317]
    tunnel: w15 -> [w316]
    tunnel: w14 -> [w315]
    tunnel: w13 -> [w314]
    tunnel: w12 -> [w313]
    tunnel: w11 -> [w312]
    tunnel: w10 -> [w311]
    tunnel: w8 -> [_]
    stop <- FALSE stop-if-true
    n159 = event shown="[11] \"写公式\": 值改变" {
      selector: _ -> [_ _ _ _ _ _ _ _ _ _ _ _ _ _ _ _]
      dyn-events: _ -> [_ _ _ _ _ _ _ _ _ _ _ _ _ _ _ _]
      timeout: _ -> [_ _ _ _ _ _ _ _ _ _ _ _ _ _ _ _]
      tunnel: w317 -> [_ _ w336 _ w347 w351 _ _ _ _ _ _ _ _ _ _]
      tunnel: w316 -> [_ _ _ _ _ _ _ _ _ _ w404 _ w424 w433 _ _]
      tunnel: w315 -> [_ _ _ _ _ _ _ _ _ _ w402 _ w422 w435 w443 w450]
      tunnel: w314 -> [_ _ _ _ _ _ _ _ _ _ w403 _ w423 w434 _ _]
      tunnel: w313 -> [_ _ _ _ _ _ _ _ _ _ w398 _ _ _ _ _]
      tunnel: w312 -> [_ _ _ _ _ _ _ _ _ _ _ _ w418 _ _ _]
      tunnel: w311 -> [_ _ _ _ _ _ _ _ _ _ _ _ _ _ w441 _]
      event Timeout {
        n160 = event-data() -> ()  [unwired: 1 in, 3 out]
      }
      event "总氮自动测试量程配置": Value Change {
        n161 = event-data() -> ()  [unwired: 1 in, 6 out]
        n162 = flat-sequence {
          frame #0 {
            n163 = global write "系统设置全局变量.vi" "总氮自动测试量程配置"("总氮自动测试量程配置") -> ()
          }
          frame #1 {
            n164 = call <vilib>:"Application Directory.vi"() -> ("Application Directory"=w333:path)
            n165 = Build Path(base path=w333, name or relative path="data\\sys.ini" ("名称或相对路径")) -> (appended path=w331:path)
            n166 = call <vilib>:"Open Config Data.vi"("configuration file path"=w331) -> ("error out"=w327:errorcluster, "refnum"=w330:T17)  [unwired: 8 in, 1 out]
            n167 = vi-ref "系统设置全局变量.vi"() -> (w329:refnum<vi>)
            n168 = call <userlib>:"Write Panel to INI__ogtk.vi"("error in (no error)"=w327, "VI ref"=w329, "refnum"=w330) -> ("error out"=w326:errorcluster, "refnum out"=w328:T17)  [unwired: 7 in]
            n169 = call <vilib>:"Close Config Data.vi"("error in (no error)"=w326, "refnum"=w328) -> ("error out"=w321:errorcluster, "file path"=w320:path)  [unwired: 8 in]
            n170 = Open/Create/Replace File(file path (use dialog)=w320, error in=w321) -> (refnum out=w324:refnum<file>, error out=w325:errorcluster)  [unwired: 4 in, 1 out]
            n171 = Flush File(refnum=w324, error in=w325) -> (refnum out=w323:refnum<file>, error out=w322:errorcluster)
            n172 = Close File(refnum=w323, error in=w322) -> ()  [unwired: 2 out]
          }
        }
      }
      event "手动启动": Value Change {
        n173 = event-data() -> ()  [unwired: 1 in, 6 out]
        n174 = call "总氮启动参数对话框.vi"() -> ("确认"=w334:bool, "元素"=w335:cluster{"命令":string, "data":variant})  [unwired: 10 in]
        n175 = case shown="真" w334 {
          tunnel: w336 -> [_ w338]
          tunnel: w335 -> [_ w337]
          frame False {
          }
          frame True {
            n176 = Enqueue Element(queue=w338, element=w337) -> ()  [unwired: 2 in, 3 out]
          }
        }
      }
      event "定时启动": Mouse Down {
        n177 = event-data() -> ()  [unwired: 1 in, 6 out]
        n178 = call "定时启动对话框.vi"() -> ("设置值"=→"设置值":dbl, "确定输出"=→"定时启动":bool)  [unwired: 10 in]
      }
      event "单步测试": Value Change {
        w342 = u16 1 items=["总磷"=1, "氨氮"=3] ("站号")
        n179 = event-data() -> ()  [unwired: 1 in, 6 out]
        n180 = Bundle("站号"=w342, "总磷氨氮调试"="总磷氨氮调试") -> (w341:cluster{"站号":u16, "总磷氨氮调试":u16[]})  [unwired: 1 in]
        n181 = Bundle By Name(cluster=cluster{"命令":string, "data":variant} {"命令"="", "data"=variant} ("元素"), "命令"="debug", "data"=w341) -> (w344:cluster{"命令":string, "data":variant})
        n182 = Enqueue Element(queue=w347, element=w344) -> ()  [unwired: 2 in, 3 out]
      }
      event "停止": Value Change {
        n183 = event-data() -> ()  [unwired: 1 in, 6 out]
        n184 = Enqueue Element(queue=w351, element=cluster{"命令":string, "data":variant} {"命令"="启动", "data"=variant(cluster{"站号":u16, "控制命令输出":u16[]} {"站号"=1, "控制命令输出"=[2816]})} ("元素")) -> (queue out=w348:refnum<queue>)  [unwired: 2 in, 2 out]
        n185 = Enqueue Element(queue=w348, element=cluster{"命令":string, "data":variant} {"命令"="启动", "data"=variant(cluster{"站号":u16, "控制命令输出":u16[]} {"站号"=2, "控制命令输出"=[2816]})} ("元素")) -> ()  [unwired: 2 in, 3 out]
      }
      event "设置": Value Change {
        n186 = event-data() -> ()  [unwired: 1 in, 6 out]
        n187 = property on="窗格" class="Pane"("Origin"=T5 {"Horizontal"=0, "Vertical"=628} ("原点")) -> ()  [unwired: 2 in, 2 out]
      }
      event "返回": Value Change {
        n188 = event-data() -> ()  [unwired: 1 in, 6 out]
        n189 = property on="窗格" class="Pane"("Origin"=T5 {"Horizontal"=0, "Vertical"=0} ("原点")) -> ()  [unwired: 2 in, 2 out]
      }
      event "标液浓度1", "测量吸光度1", "测量吸光度2", "标液浓度2", "测量吸光度3", "标液浓度3", "测量吸光度4", "标液浓度4", "测量吸光度5", "标液浓度5", "样品1启用", "样品3启用", "样品4启用", "样品5启用", "样品2启用", "模型", "method", "样品1 F0", "样品1 F1", "样品2 F1", "样品2 F0", "样品3 F1", "样品4 F0", "样品4 F1", "样品5 F1", "样品5 F0", "精度": Value Change {
        n190 = event-data() -> ()  [unwired: 1 in, 6 out]
        n191 = formula code="E=log(F0/F1);"("F0"="样品1 F0", "F1"="样品1 F1") -> ("E"=w375:dbl)
        "测量吸光度1" <- w375
        n192 = formula code="E=log(F0/F1);"("F0"="样品2 F0", "F1"="样品2 F1") -> ("E"=w372:dbl)
        "测量吸光度2" <- w372
        n193 = formula code="E=log(F0/F1);"("F0"="样品3 F0", "F1"="样品3 F1") -> ("E"=w369:dbl)
        "测量吸光度3" <- w369
        n194 = formula code="E=log(F0/F1);"("F0"="样品4 F0", "F1"="样品4 F1") -> ("E"=w366:dbl)
        "测量吸光度4" <- w366
        n195 = formula code="E=log(F0/F1);"("F0"="样品5 F0", "F1"="样品5 F1") -> ("E"=w363:dbl)
        "测量吸光度5" <- w363
        n196 = Replace Array Subset(array=dbl[] [0.0, 0.0, 0.0, 0.0, 0.0] ("数组"), new element #1="标液浓度1", new element #2="标液浓度2", new element #3="标液浓度3", new element #4="标液浓度4", new element #5="标液浓度5") -> (w360:dbl[])  [unwired: 5 in]
        n197 = Replace Array Subset(array=dbl[] [0.0, 0.0, 0.0, 0.0, 0.0] ("数组"), new element #1=w375, new element #2=w372, new element #3=w369, new element #4=w366, new element #5=w363) -> (w359:dbl[])  [unwired: 5 in]
        n198 = Replace Array Subset(array=bool[] [FALSE, FALSE, FALSE, FALSE, FALSE] ("数组"), new element #1="样品1启用", new element #2="样品2启用", new element #3="样品3启用", new element #4="样品4启用", new element #5="样品5启用") -> (w358:bool[])  [unwired: 5 in]
        n199 = call "线性公式.vi"("精度"="精度", "模型"="模型", "method"="method", "启用"=w358, "监测浓度"=w359, "标液浓度"=w360) -> ("XY图"=→"XY图":cluster{"X Values":dbl[], "Y Values":dbl[]}[], "r^2"=→"r^2":dbl, "拟合方程"=→"拟合公式":string)  [unwired: 3 in]
      }
      event "标液浓度1", "标液浓度2", "标液浓度3", "标液浓度4", "标液浓度5", "样品1 F0", "样品1 F1", "样品2 F1", "样品2 F0", "样品3 F1", "样品3 F0", "样品4 F0", "样品4 F1", "样品5 F0", "样品5 F1", "精度", "公式.X^2", "公式.X", "公式.b", "量程切换阈值.阈值", "量程切换阈值.标液浓度", "备用系数.量程上限", "备用系数.量程下限", "备用系数.检出限", "备用系数.精度": Mouse Down {
        n200 = event-data() -> ("CtlRef"=w394:refnum<vi>)  [unwired: 1 in, 5 out]
        n201 = property class="DigNum (严格)"(reference=w394) -> (reference out=w392:refnum<vi>, "Value"=w393:dbl)  [unwired: 1 in, 1 out]
        n202 = call "数字键盘.vi"("OldNumber"=w393) -> ("NewNumber"=w391:sgl)
        n203 = property class="DigNum (严格)"(reference=w392, "Val(Sgnl)"=w391) -> ()  [unwired: 1 in, 2 out]
      }
      event "读公式": Value Change {
        n204 = event-data() -> ()  [unwired: 1 in, 6 out]
        n205 = property class="Enum (严格)"(reference=w402) -> ("Value"=w401:enum16{"总磷", "总氮"})  [unwired: 1 in, 2 out]
        n206 = property class="Enum (严格)"(reference=w403) -> ("Value"=w400:enum16{"水样测量", "空白核查", "跨度核查", "标样核查", "加标回收"})  [unwired: 1 in, 2 out]
        n207 = property class="Enum (严格)"(reference=w404) -> ("Value"=w399:enum16{"低量程", "高量程"})  [unwired: 1 in, 2 out]
        n208 = call "总氮公式读取.vi"("量程"=w399, "测量模式"=w400, "测量参数"=w401) -> ("error out"=w396:errorcluster, "公式"=w397:cluster{"X^2":dbl, "X":dbl, "b":dbl})  [unwired: 7 in]
        n209 = property class="Clust (严格)"(reference=w398, "Value"=w397) -> ()  [unwired: 1 in, 2 out]
        n210 = case shown="错误" w396 {
          tunnel: ["读取成功" ("消息") "读取失败" ("消息")] -> w395
          frame No Error {
          }
          frame Error {
          }
        }
        n211 = One Button Dialog(message=w395) -> ()  [unwired: 1 in, 1 out]
      }
      event "写公式": Value Change {
        n212 = event-data() -> ()  [unwired: 1 in, 6 out]
        n213 = call "总氮公式写入.vi"("公式"="公式", "量程"="量程下拉列表", "测量模式"="测量模式下拉列表", "测量参数"="参数下拉列表") -> ("error out"=w409:errorcluster)  [unwired: 7 in]
        n214 = case shown="无错误" w409 {
          tunnel: ["写入成功" ("消息") "写入失败" ("消息")] -> w410
          frame No Error {
          }
          frame Error {
          }
        }
        n215 = One Button Dialog(message=w410) -> ()  [unwired: 1 in, 1 out]
      }
      event "量程切换阈值读取": Value Change {
        n216 = event-data() -> ()  [unwired: 1 in, 6 out]
        n217 = property class="Enum (严格)"(reference=w422) -> ("Value"=w421:enum16{"总磷", "总氮"})  [unwired: 1 in, 2 out]
        n218 = property class="Enum (严格)"(reference=w423) -> ("Value"=w420:enum16{"水样测量", "空白核查", "跨度核查", "标样核查", "加标回收"})  [unwired: 1 in, 2 out]
        n219 = property class="Enum (严格)"(reference=w424) -> ("Value"=w419:enum16{"低量程", "高量程"})  [unwired: 1 in, 2 out]
        n220 = call "总氮量程读取.vi"("量程"=w419, "测量模式"=w420, "测量参数"=w421) -> ("error out"=w415:errorcluster, "量程切换阈值"=w417:cluster{"阈值":dbl, "标液浓度":dbl})  [unwired: 7 in]
        n221 = property class="Clust (严格)"(reference=w418, "Value"=w417) -> ()  [unwired: 1 in, 2 out]
        n222 = case shown="错误" w415 {
          tunnel: ["读取成功" ("消息") "读取失败" ("消息")] -> w416
          frame No Error {
          }
          frame Error {
          }
        }
        n223 = One Button Dialog(message=w416) -> ()  [unwired: 1 in, 1 out]
      }
      event "量程切换阈值写入": Value Change {
        n224 = event-data() -> ()  [unwired: 1 in, 6 out]
        n225 = property class="Enum (严格)"(reference=w435) -> ("Value"=w432:enum16{"总磷", "总氮"})  [unwired: 1 in, 2 out]
        n226 = property class="Enum (严格)"(reference=w434) -> ("Value"=w431:enum16{"水样测量", "空白核查", "跨度核查", "标样核查", "加标回收"})  [unwired: 1 in, 2 out]
        n227 = property class="Enum (严格)"(reference=w433) -> ("Value"=w430:enum16{"低量程", "高量程"})  [unwired: 1 in, 2 out]
        n228 = call "总氮量程写入.vi"("量程切换阈值"="量程切换阈值", "量程"=w430, "测量模式"=w431, "测量参数"=w432) -> ("error out"=w427:errorcluster)  [unwired: 7 in]
        n229 = case shown="无错误" w427 {
          tunnel: ["写入成功" ("消息") "写入失败" ("消息")] -> w428
          frame No Error {
          }
          frame Error {
          }
        }
        n230 = One Button Dialog(message=w428) -> ()  [unwired: 1 in, 1 out]
      }
      event "备用系数读取": Value Change {
        n231 = event-data() -> ()  [unwired: 1 in, 6 out]
        n232 = property class="Enum (严格)"(reference=w443) -> ("Value"=w442:enum16{"总磷", "总氮"})  [unwired: 1 in, 2 out]
        n233 = call "总氮备用系数读取.vi"("测量参数"=w442) -> ("error out"=w438:errorcluster, "备用系数"=w440:T2)  [unwired: 9 in]
        n234 = property class="Clust (严格)"(reference=w441, "Value"=w440) -> ()  [unwired: 1 in, 2 out]
        n235 = case shown="错误" w438 {
          tunnel: ["读取成功" ("消息") "读取失败" ("消息")] -> w439
          frame No Error {
          }
          frame Error {
          }
        }
        n236 = One Button Dialog(message=w439) -> ()  [unwired: 1 in, 1 out]
      }
      event "备用系数写入": Value Change {
        n237 = event-data() -> ()  [unwired: 1 in, 6 out]
        n238 = property class="Enum (严格)"(reference=w450) -> ("Value"=w449:enum16{"总磷", "总氮"})  [unwired: 1 in, 2 out]
        n239 = call "总氮备用系数写入.vi"("备用系数"="备用系数", "测量参数"=w449) -> ("error out"=w446:errorcluster)  [unwired: 9 in]
        n240 = case shown="无错误" w446 {
          tunnel: ["写入成功" ("消息") "写入失败" ("消息")] -> w447
          frame No Error {
          }
          frame Error {
          }
        }
        n241 = One Button Dialog(message=w447) -> ()  [unwired: 1 in, 1 out]
      }
    }
  }
  n242 = call-by-ref "?"(reference=w29, error in=w27) -> (reference out=w25:refnum<vi>, error out=w26:errorcluster)  [unwired: 12 in]
  n243 = Open VI Reference(type specifier VI Refnum (for type only)=refnum<vi> refnum, vi path=w17, options=128 ("选项")) -> (vi reference=w19:refnum<vi>, error out=w21:errorcluster)  [unwired: 3 in]
  n244 = call-by-ref "?"(reference=w19, error in=w21) -> (reference out=w23:refnum<vi>, error out=w22:errorcluster)  [unwired: 12 in]
  n245 = Close Reference(reference=w25, error in (no error)=w26) -> ()  [unwired: 1 out]
  n246 = Close Reference(reference=w23, error in (no error)=w22) -> ()  [unwired: 1 out]
  n247 = while {
    tunnel: w35 -> [w457]
    shift-right: [w458] -> _
    shift-left: enum16{"待机", "启动", "测量中", "延时"}."待机" -> [w459]
    shift-right: [w455] -> _
    shift-left: u32 0 ("等待时间（毫秒）") -> [w456]
    stop <- FALSE stop-if-true
    n248 = Wait (ms)(milliseconds to wait=u32 1000 ("等待时间（毫秒）")) -> ()  [unwired: 1 out]
    n249 = local read "定时启动"() -> (w460:bool)
    n250 = global read "系统设置全局变量.vi" "总氮自动测试量程配置"() -> (w453:T1)
    n251 = case shown="真" w460 {
      tunnel: w459 -> [_ w469]
      tunnel: [enum16{"待机", "启动", "测量中", "延时"}."待机" w468] -> w458
      tunnel: w457 -> [_ w467]
      tunnel: w456 -> [_ w466]
      tunnel: [_ w465] -> w455
      tunnel: [_ w464] -> w454
      frame False {
      }
      frame True {
        n252 = case shown="\"启动\"" w469 {
          tunnel: [enum16{"待机", "启动", "测量中", "延时"}."待机" w483 w509 w527] -> w468
          tunnel: w467 -> [_ w487 _ _]
          tunnel: w466 -> [_ w473 _ w518]
          tunnel: [_ w474 _ w523] -> w465
          tunnel: ["待机" ("字符串") "启动总氮" ("字符串") "总氮运行中" ("字符串") w521] -> w464
          frame "待机", Default {
          }
          frame "启动" {
            n253 = Equal To 0?(x=w473) -> (x = 0?=w472:bool)
            n254 = case shown="真" w472 {
              frame False {
              }
              frame True {
                n255 = global read "VAR总氮全局变量.vi" "总氮测量数据区"() -> (w506:T6)
                n256 = global read "VAR总氮全局变量.vi" "状态告警区"() -> (w507:T4)
                n257 = Unbundle By Name(w507) -> ("id"=w496:u16, "flowid"=w495:u16, "量程"=w494:u16)
                n258 = Unbundle By Name(w506) -> ("F0"=w505:sgl, "F1"=w504:sgl, "F2"=w503:sgl, "F3"=w502:sgl, "F4"=w501:sgl, "F5"=w500:sgl, "F6"=w499:sgl, "F7"=w498:sgl, "X值"=w497:sgl)
                n259 = Format Into String(format string="F0=%#f,F1=%#f,F2=%#f,F3=%#f,F4=%#f,F5=%#f,F6=%#f,F7=%#f,X=%#f,Flow=%d-%d-%d" ("格式字符串"), w505, w504, w503, w502, w501, w500, w499, w498, w497, w496, w495, w494) -> (resulting string=w488:string)  [unwired: 2 in, 1 out]
                n260 = Get Date/Time In Seconds() -> (seconds since 1Jan1904=w492:timestamp)
                n261 = Bundle By Name(cluster=T12 {"时间标识"=timestamp(0 s since 1904-01-01), "设备"="", "日志信息"="", "流程参数"=""} ("data in"), "时间标识"=w492, "设备"="总氮", "日志信息"="-->>总氮启动" ("设备"), "流程参数"=w488) -> (w493:T12)
                n262 = call "总氮操作日志.vi"("data in"=w493) -> ()  [unwired: 11 in]
              }
            }
            n263 = global read "系统设置全局变量.vi" "总氮自动测试量程配置"() -> (w478:T1)
            n264 = Unbundle By Name(w478) -> ("水样测试量程模式"=w477:enum16{"H", "L", "AUTO"})
            n265 = Bundle By Name(cluster=T16 {"站号"=2, "量程切换"=enum."AUTO", "控制命令"=enum."启动测量", "模式设置"=enum."待机", "测量间隔"=0} ("参数"), "量程切换"=w477) -> (w475:T16)
            n266 = call "总氮启动命令.vi"("参数"=w475) -> ("启动命令"=w481:cluster{"命令":string, "data":variant})  [unwired: 10 in]
            n267 = Enqueue Element(queue=w487, element=w481) -> ()  [unwired: 2 in, 3 out]
            n268 = Increment(x=w473) -> (x+1=w474:u32)
            n269 = global read "VAR总氮全局变量.vi" "状态告警区"() -> (w486:T4)
            n270 = Unbundle By Name(w486) -> ("工作状态"=w485:T7)
            n271 = Not Equal To 0?(x=w485) -> (x != 0?=w484:bool)
            n272 = Select(t=enum16{"待机", "启动", "测量中", "延时"}."测量中", s=w484, f=enum16{"待机", "启动", "测量中", "延时"}."启动") -> (s? t:f=w483:enum16{"待机", "启动", "测量中", "延时"})
          }
          frame "测量中" {
            n273 = global read "VAR总氮全局变量.vi" "状态告警区"() -> (w512:T4)
            n274 = Unbundle By Name(w512) -> ("工作状态"=w510:T7, "id"=w511:u16)
            n275 = case shown="\"空闲\"" w510 {
              tunnel: w511 -> [_ _]
              tunnel: [enum16{"待机", "启动", "测量中", "延时"}."启动" enum16{"待机", "启动", "测量中", "延时"}."测量中"] -> w509
              frame "空闲" {
                n276 = Wait (ms)(milliseconds to wait=u32 8000 ("等待时间（毫秒）")) -> ()  [unwired: 1 out]
              }
              frame Default {
              }
            }
          }
          frame "延时" {
            n277 = Equal To 0?(x=w518) -> (x = 0?=w517:bool)
            n278 = case shown="真" w517 {
              frame False {
              }
              frame True {
                n279 = global read "VAR总氮全局变量.vi" "总氮测量数据区"() -> (w547:T6)
                n280 = global read "VAR总氮全局变量.vi" "状态告警区"() -> (w548:T4)
                n281 = Unbundle By Name(w548) -> ("id"=w537:u16, "flowid"=w536:u16, "量程"=w535:u16)
                n282 = Unbundle By Name(w547) -> ("F0"=w546:sgl, "F1"=w545:sgl, "F2"=w544:sgl, "F3"=w543:sgl, "F4"=w542:sgl, "F5"=w541:sgl, "F6"=w540:sgl, "F7"=w539:sgl, "X值"=w538:sgl)
                n283 = Format Into String(format string="F0=%#f,F1=%#f,F2=%#f,F3=%#f,F4=%#f,F5=%#f,F6=%#f,F7=%#f,X=%#f,Flow=%d-%d-%d" ("格式字符串"), w546, w545, w544, w543, w542, w541, w540, w539, w538, w537, w536, w535) -> (resulting string=w529:string)  [unwired: 2 in, 1 out]
                n284 = Get Date/Time In Seconds() -> (seconds since 1Jan1904=w533:timestamp)
                n285 = Bundle By Name(cluster=T12 {"时间标识"=timestamp(0 s since 1904-01-01), "设备"="", "日志信息"="", "流程参数"=""} ("data in"), "时间标识"=w533, "设备"="总氮", "日志信息"="-->>总氮停止" ("设备"), "流程参数"=w529) -> (w534:T12)
                n286 = call "总氮操作日志.vi"("data in"=w534) -> ()  [unwired: 11 in]
              }
            }
            n287 = local read "设置值"() -> (w526:dbl)
            n288 = Increment(x=w518) -> (x+1=w523:u32)
            n289 = Add(x=w526, y=10.0) -> (x+y=w524:dbl)
            n290 = Greater Or Equal?(x=w523, y=w524) -> (x >= y?=w528:bool)
            n291 = Select(t=enum16{"待机", "启动", "测量中", "延时"}."待机", s=w528, f=enum16{"待机", "启动", "测量中", "延时"}."延时") -> (s? t:f=w527:enum16{"待机", "启动", "测量中", "延时"})
            n292 = Format Into String(format string="延时计时中%d秒" ("格式字符串"), w523) -> (resulting string=w521:string)  [unwired: 2 in, 1 out]
          }
        }
      }
    }
    "字符串" <- w454
    n293 = local write "总氮自动测试量程配置"(w453) -> ()
  }
  n294 = node-c288(w5) -> ()  [unwired: 1 out]
